vi "Lab Panel V2.5.vi"() -> ()   [LabVIEW 2013]
uses:
  <vilib>/Platform/TimedLoop/XDataNode/timing_clust.ctl
  <vilib>/Platform/TimedLoop/XDataNode/nitl_modes.ctl
  <vilib>/Platform/TimedLoop/XDataNode/wakeup.ctl
  <vilib>/platform/TimedLoop/XDataNode/XDataNode.xnode
  <vilib>/Platform/TimedLoop/XDataNode/XDNodeRunTimeDep.lvlib
panel:
  out "TEMP update":bool
  out "AI update":bool
  in  "stop":bool
  in  "Tab Control 2":T1(tab)
  out "LAB05-2 (SIG)":T2 {"PF" format="%.2f"; "AMPS" format="%.1f"}
  out "LAB05-1 (SIG)":T2 {"PF" format="%.2f"; "AMPS" format="%.1f"}
  out "LAB04-2 (SIG)":T2 {"PF" format="%.2f"; "AMPS" format="%.1f"}
  out "LAB04-1 (SIG)":T2 {"PF" format="%.2f"; "AMPS" format="%.1f"}
  out "LAB03-2 (SIG)":T2 {"PF" format="%.2f"; "AMPS" format="%.1f"}
  out "LAB03-1 (SIG)":T2 {"PF" format="%.2f"; "AMPS" format="%.1f"}
  out "LAB02-2 (SIG)":T2 {"PF" format="%.2f"; "AMPS" format="%.1f"}
  in  "LAB01-1RUN":bool
  in  "LAB05-1 (O/I)":bool
  in  "LAB05-2 (O/I)":bool
  in  "LAB04-1 (O/I)":bool
  in  "LAB04-2 (O/I)":bool
  in  "LAB02-1 (O/I)":bool
  in  "LAB02-2 (O/I)":bool
  in  "LAB01-2 (O/I)":bool
  in  "LAB01-1 (O/I)":bool
  in  "LAB03-1 (O/I)":bool
  in  "LAB05-2 RUN":bool
  in  "LAB05-1 RUN":bool
  in  "LAB04-2 RUN":bool
  in  "LAB04-1 RUN":bool
  in  "LAB03-2 RUN":bool
  in  "LAB03-1 RUN":bool
  in  "LAB02-2 RUN":bool
  in  "LAB02-1 RUN":bool
  in  "LAB01-2 RUN":bool
  in  "LAB05-2 SELECT":T3(radio)
  in  "LAB05-1 SELECT":T3(radio)
  in  "LAB04-2 SELECT":T3(radio)
  in  "LAB04-1 SELECT":T3(radio)
  in  "LAB03-2 SELECT":T3(radio)
  in  "LAB03-1 SELECT":T3(radio)
  in  "LAB02-2 SELECT":T3(radio)
  in  "LAB02-1 SELECT":T3(radio)
  in  "LAB01-2 SELECT":T3(radio)
  in  "LAB01-1 SELECT":T3(radio)
  in  "LAB03-2 (O/I)":bool
  out "LAB01-1 (SIG)":T2 {"PF" format="%.2f"; "AMPS" format="%.1f"}
  out "LAB01-2 (SIG)":T2 {"PF" format="%.2f"; "AMPS" format="%.1f"}
  out "LAB02-1 (SIG)":T2 {"PF" format="%.2f"; "AMPS" format="%.1f"}
  out "LAB05-2 (RESULT)":bool
  out "LAB05-1 (RESULT)":bool
  out "LAB04-2 (RESULT)":bool
  out "LAB04-1 (RESULT)":bool
  out "LAB03-2 (RESULT)":bool
  out "LAB03-1 (RESULT)":bool
  out "LAB02-2 (RESULT)":bool
  out "LAB02-1 (RESULT)":bool
  out "LAB01-2 (RESULT)":bool
  out "LAB01-1 (RESULT)":bool
  in  "LAB05 (SET)":T4={"1 Name"="", "1 Description"="", "1 (CYCLES)"=1.0, "1 (T-RISE mins)"=1.0, "1 (T-RISE deg C)"=1.0, "2 Name"="", "2 Description"="", "2 (CYCLES)"=1.0, "2 (T-RISE mins)"=1.0, "2 (T-RISE deg C)"=1.0} {"2 (T-RISE deg C)" min=1.0 max=100.0 step=1.0 format="%#.0f"; "2 (T-RISE mins)" min=0.0 max=1000.0 step=10.0 format="%#.0f"; "2 (CYCLES)" min=0.0 max=100000.0 step=10.0; "1 (T-RISE deg C)" min=1.0 max=100.0 step=1.0 format="%#.0f"; "1 (T-RISE mins)" min=0.0 max=1000.0 step=10.0 format="%#.0f"; "1 (CYCLES)" min=0.0 max=100000.0 step=10.0}
  in  "LAB04 (SET)":T4={"1 Name"="", "1 Description"="", "1 (CYCLES)"=1.0, "1 (T-RISE mins)"=1.0, "1 (T-RISE deg C)"=1.0, "2 Name"="", "2 Description"="", "2 (CYCLES)"=1.0, "2 (T-RISE mins)"=1.0, "2 (T-RISE deg C)"=1.0} {"2 (T-RISE deg C)" min=1.0 max=100.0 step=1.0 format="%#.0f"; "2 (T-RISE mins)" min=0.0 max=1000.0 step=10.0 format="%#.0f"; "2 (CYCLES)" min=0.0 max=100000.0 step=10.0; "1 (T-RISE deg C)" min=1.0 max=100.0 step=1.0 format="%#.0f"; "1 (T-RISE mins)" min=0.0 max=1000.0 step=10.0 format="%#.0f"; "1 (CYCLES)" min=0.0 max=100000.0 step=10.0}
  in  "LAB03 (SET)":T4={"1 Name"="", "1 Description"="", "1 (CYCLES)"=1.0, "1 (T-RISE mins)"=1.0, "1 (T-RISE deg C)"=1.0, "2 Name"="", "2 Description"="", "2 (CYCLES)"=1.0, "2 (T-RISE mins)"=1.0, "2 (T-RISE deg C)"=1.0} {"2 (T-RISE deg C)" min=1.0 max=100.0 step=1.0 format="%#.0f"; "2 (T-RISE mins)" min=0.0 max=1000.0 step=10.0 format="%#.0f"; "2 (CYCLES)" min=0.0 max=100000.0 step=10.0; "1 (T-RISE deg C)" min=1.0 max=100.0 step=1.0 format="%#.0f"; "1 (T-RISE mins)" min=0.0 max=1000.0 step=10.0 format="%#.0f"; "1 (CYCLES)" min=0.0 max=100000.0 step=10.0}
  out "LAB05 (DISP)":T5 {"2 (T-RISE min)" format="%#.0f"; "2 (CYCLE)" format="%#.0f"; "1 (T-RISE min)" format="%#.0f"; "1 (CYCLE)" format="%#.0f"}
  out "LAB04 (DISP)":T5 {"2 (T-RISE min)" format="%#.0f"; "2 (CYCLE)" format="%#.0f"; "1 (T-RISE min)" format="%#.0f"; "1 (CYCLE)" format="%#.0f"}
  out "LAB03 (DISP)":T5 {"2 (T-RISE min)" format="%#.0f"; "2 (CYCLE)" format="%#.0f"; "1 (T-RISE min)" format="%#.0f"; "1 (CYCLE)" format="%#.0f"}
  out "LAB02 (DISP)":T5 {"2 (T-RISE min)" format="%#.0f"; "2 (CYCLE)" format="%#.0f"; "1 (T-RISE min)" format="%#.0f"; "1 (CYCLE)" format="%#.0f"}
  in  "LAB02 (SET)":T4={"1 Name"="", "1 Description"="", "1 (CYCLES)"=1.0, "1 (T-RISE mins)"=1.0, "1 (T-RISE deg C)"=1.0, "2 Name"="", "2 Description"="", "2 (CYCLES)"=1.0, "2 (T-RISE mins)"=1.0, "2 (T-RISE deg C)"=1.0} {"2 (T-RISE deg C)" min=1.0 max=100.0 step=1.0 format="%#.0f"; "2 (T-RISE mins)" min=0.0 max=1000.0 step=10.0 format="%#.0f"; "2 (CYCLES)" min=0.0 max=100000.0 step=10.0; "1 (T-RISE deg C)" min=1.0 max=100.0 step=1.0 format="%#.0f"; "1 (T-RISE mins)" min=0.0 max=1000.0 step=10.0 format="%#.0f"; "1 (CYCLES)" min=0.0 max=100000.0 step=10.0}
  out "LAB01 (DISP)":T5 {"2 (T-RISE min)" format="%#.0f"; "2 (CYCLE)" format="%#.0f"; "1 (T-RISE min)" format="%.2f"; "1 (CYCLE)" format="%#.0f"}
  in  "LAB01 (SET)":T4={"1 Name"="", "1 Description"="", "1 (CYCLES)"=1.0, "1 (T-RISE mins)"=1.0, "1 (T-RISE deg C)"=1.0, "2 Name"="", "2 Description"="", "2 (CYCLES)"=1.0, "2 (T-RISE mins)"=1.0, "2 (T-RISE deg C)"=1.0} {"2 (T-RISE deg C)" min=1.0 max=100.0 step=1.0 format="%#.0f"; "2 (T-RISE mins)" min=1.0 max=1000.0 step=10.0 format="%#.0f"; "2 (CYCLES)" min=1.0 max=100000.0 step=10.0; "1 (T-RISE deg C)" min=1.0 max=100.0 step=1.0 format="%#.0f"; "1 (T-RISE mins)" min=1.0 max=1000.0 step=10.0 format="%#.0f"; "1 (CYCLES)" min=1.0 max=100000.0 step=10.0}
  out "LAB05 (TEMP START)":T6
  out "LAB04 (TEMP START)":T6
  out "LAB03 (TEMP START)":T6
  out "LAB02 (TEMP START)":T6
  out "LAB01 (TEMP START)":T6
  in  "JIG ON TIME (S)":dbl=1.0 min=1.0 max=10.0 step=0.5 format="%.1g"
  in  "JIG OFF TIME (S)":dbl=2.0 min=2.0 max=10.0 step=0.5 format="%.1g"
  out "LAB01-1 (JIG)":bool
  out "LAB01-2 (JIG)":bool
  out "LAB02-1 (JIG)":bool
  out "LAB02-2 (JIG)":bool
  out "LAB03-1 (JIG)":bool
  out "LAB03-2 (JIG)":bool
  out "LAB04-1 (JIG)":bool
  out "LAB04-2 (JIG)":bool
  out "LAB05-1 (JIG)":bool
  out "LAB05-2 (JIG)":bool
  out "LAB01 (CAL)":T7 {"2 (TN) cal" min=0.0 step=0.01 format="%.2f"; "2 (TL) cal" min=0.0 step=0.01 format="%.2f"; "2 (PF) cal" min=0.0 step=0.01 format="%.2f"; "2 (V) cal" min=0.0 step=0.01 format="%.2f"; "2 (A) cal" min=0.0 step=0.01 format="%.2f"; "1 (TN) cal" min=0.0 step=0.01 format="%.2f"; "1 (TL) cal" min=0.0 step=0.01 format="%.2f"; "1 (PF) cal" min=0.0 step=0.01 format="%.2f"; "1 (V) cal" min=0.0 step=0.01 format="%.2f"; "1  (A) cal" min=0.0 step=0.01 format="%.2f"}
  out "LAB03 (CAL)":T7 {"2 (TN) cal" min=0.0 step=0.01 format="%.2f"; "2 (TL) cal" min=0.0 step=0.01 format="%.2f"; "2 (PF) cal" min=0.0 step=0.01 format="%.2f"; "2 (V) cal" min=0.0 step=0.01 format="%.2f"; "2 (A) cal" min=0.0 step=0.01 format="%.2f"; "1 (TN) cal" min=0.0 step=0.01 format="%.2f"; "1 (TL) cal" min=0.0 step=0.01 format="%.2f"; "1 (PF) cal" min=0.0 step=0.01 format="%.2f"; "1 (V) cal" min=0.0 step=0.01 format="%.2f"; "1  (A) cal" min=0.0 step=0.01 format="%.2f"}
  out "LAB02 (CAL)":T8 {"2 (TN) cal" min=0.0 step=0.01 format="%.2f"; "2 (TL) cal" min=0.0 step=0.01 format="%.2f"; "2 (PF) cal" min=0.0 step=0.01 format="%.2f"; "2 (V) cal" min=0.0 step=0.01 format="%.2f"; "2 (A) cal" min=0.0 step=0.01 format="%.2f"; "1 (TN) cal" min=0.0 step=0.01 format="%.2f"; "1 (TL) cal" min=0.0 step=0.01 format="%.2f"; "1 (PF) cal" min=0.0 step=0.01 format="%.2f"; "1 (V) cal" min=0.0 step=0.01 format="%.2f"; "1 (A) cal" min=0.0 step=0.01 format="%.2f"}
  out "LAB05 (CAL)":T7 {"2 (TN) cal" min=0.0 step=0.01 format="%.2f"; "2 (TL) cal" min=0.0 step=0.01 format="%.2f"; "2 (PF) cal" min=0.0 step=0.01 format="%.2f"; "2 (V) cal" min=0.0 step=0.01 format="%.2f"; "2 (A) cal" min=0.0 step=0.01 format="%.2f"; "1 (TN) cal" min=0.0 step=0.01 format="%.2f"; "1 (TL) cal" min=0.0 step=0.01 format="%.2f"; "1 (PF) cal" min=0.0 step=0.01 format="%.2f"; "1 (V) cal" min=0.0 step=0.01 format="%.2f"; "1  (A) cal" min=0.0 step=0.01 format="%.2f"}
  out "LAB04 (CAL)":T7 {"2 (TN) cal" min=0.0 step=0.01 format="%.2f"; "2 (TL) cal" min=0.0 step=0.01 format="%.2f"; "2 (PF) cal" min=0.0 step=0.01 format="%.2f"; "2 (V) cal" min=0.0 step=0.01 format="%.2f"; "2 (A) cal" min=0.0 step=0.01 format="%.2f"; "1 (TN) cal" min=0.0 step=0.01 format="%.2f"; "1 (TL) cal" min=0.0 step=0.01 format="%.2f"; "1 (PF) cal" min=0.0 step=0.01 format="%.2f"; "1 (V) cal" min=0.0 step=0.01 format="%.2f"; "1  (A) cal" min=0.0 step=0.01 format="%.2f"}
  out "calibration file error out":errorcluster
  in  "CALIBRATE":bool
  in  "Tab Control":T9(tab)
  out "LAB01-2 (GRAPH)":dynamicdata(graph)
  out "LAB01-1 (GRAPH)":dynamicdata(graph)
  out "LAB02-2 (GRAPH)":dynamicdata(graph)
  out "LAB02-1 (GRAPH)":dynamicdata(graph)
  out "LAB03-2 (GRAPH)":dynamicdata(graph)
  out "LAB03-1 (GRAPH)":dynamicdata(graph)
  out "LAB04-2 (GRAPH)":dynamicdata(graph)
  out "LAB04-1 (GRAPH)":dynamicdata(graph)
  out "LAB05-2 (GRAPH)":dynamicdata(graph)
  out "LAB05-1 (GRAPH)":dynamicdata(graph)
  out "LAB05 TEMP":T10
  out "LAB04 TEMP":T10
  out "LAB02 TEMP":T10
  out "LAB01 TEMP":T10
  out "LAB03 TEMP":T10
  out "Analog Error Array":errorcluster[](array[cluster])
  out "AI loop time":dbl format="%.6g"
  out "loops":dbl
  in  "loop  delay(mS)":dbl
  out "on loops":dbl
  out "off loops":dbl
  out "jig cycle":dbl
  out "LAB01-1 (TDMS)":refnum<k34>
  out "data file error":errorcluster
  out "LAB01-2 (TDMS)":refnum<k34>
  out "LAB02-1 (TDMS)":refnum<k34>
  out "LAB02-2 (TDMS)":refnum<k34>
  out "LAB03-1 (TDMS)":refnum<k34>
  out "LAB03-2 (TDMS)":refnum<k34>
  out "LAB04-1 (TDMS)":refnum<k34>
  out "LAB04-2 (TDMS)":refnum<k34>
  out "LAB05-1 (TDMS)":refnum<k34>
  out "LAB05-2 (TDMS)":refnum<k34>
  # "LAB01"
  # "LAB02"
  # "LAB05"
  # "LAB03"
  # "LAB04"
  # "LAB01"
  # "LAB02"
  # "LAB03"
  # "LAB04"
  # "LAB05"
  # "JIG SET"
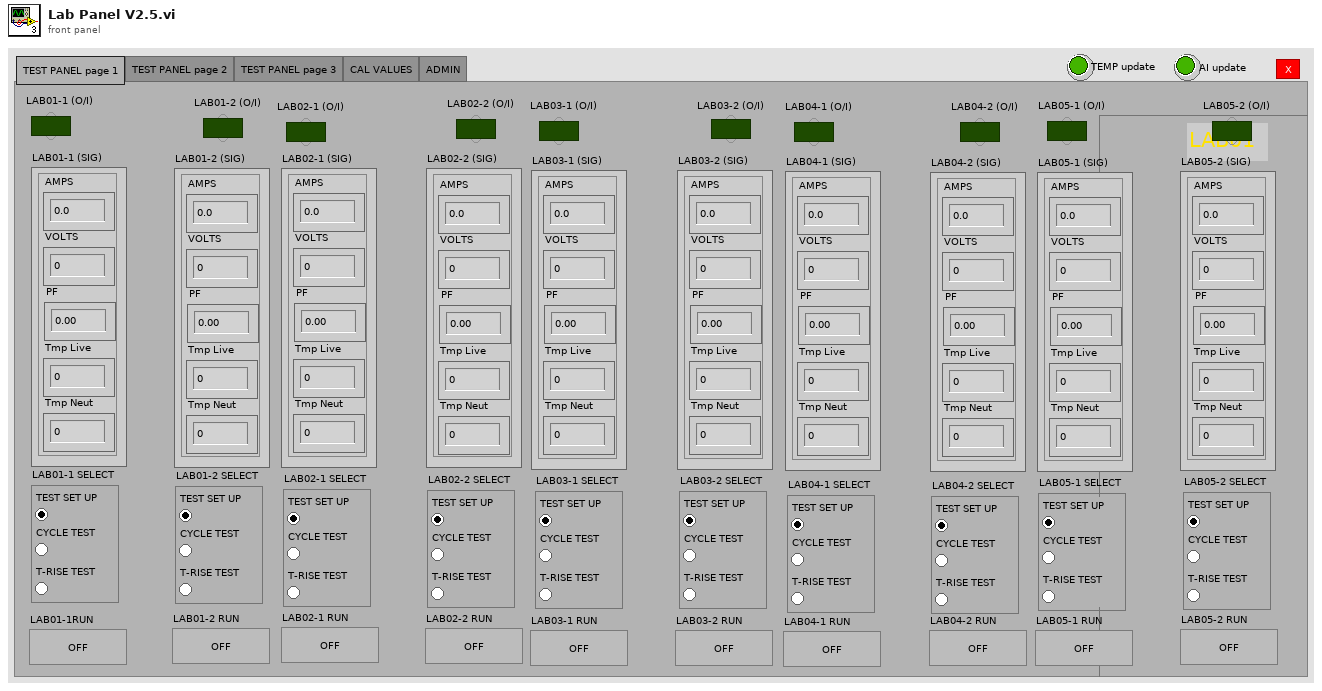
[diagram p1: front panel]
types:
  T1 = enum32{"TEST PANEL page 1", "TEST PANEL page 2", "TEST PANEL page 3", "CAL VALUES", "ADMIN"}
  T2 = cluster{"AMPS":dbl, "VOLTS":dbl, "PF":dbl, "Tmp Live":dbl, "Tmp Neut":dbl}
  T3 = enum32{"TEST SET UP", "CYCLE TEST", "T-RISE TEST"}
  T4 = cluster{"1 Name":string, "1 Description":string, "1 (CYCLES)":dbl, "1 (T-RISE mins)":dbl, "1 (T-RISE deg C)":dbl, "2 Name":string, "2 Description":string, "2 (CYCLES)":dbl, "2 (T-RISE mins)":dbl, "2 (T-RISE deg C)":dbl}
  T5 = cluster{"1 (CYCLE)":dbl, "1 (T-RISE min)":dbl, "1 (STATUS)":string, "2 (CYCLE)":dbl, "2 (T-RISE min)":dbl, "2 (STATUS)":string}
  T6 = cluster{"1 (TL)":dbl, "1 (TN)":dbl, "2 (TL)":dbl, "2 (TN)":dbl}
  T7 = cluster{"1  (A) cal":dbl, "1 (V) cal":dbl, "1 (PF) cal":dbl, "1 (TL) cal":dbl, "1 (TN) cal":dbl, "2 (A) cal":dbl, "2 (V) cal":dbl, "2 (PF) cal":dbl, "2 (TL) cal":dbl, "2 (TN) cal":dbl}
  T8 = cluster{"1 (A) cal":dbl, "1 (V) cal":dbl, "1 (PF) cal":dbl, "1 (TL) cal":dbl, "1 (TN) cal":dbl, "2 (A) cal":dbl, "2 (V) cal":dbl, "2 (PF) cal":dbl, "2 (TL) cal":dbl, "2 (TN) cal":dbl}
  T9 = enum32{"LAB01", "LAB02", "LAB03", "LAB04", "LAB05", "TEMPERATURE", "ERROR"}
  T10 = cluster{"T1 Live":dbl, "T1 Neut":dbl, "T2 Live":dbl, "T2 Neut":dbl, "ID":dbl, "ER":dbl}
  T11 = typedef "XDNodeRunTimeDep.lvlib/timing_clust.ctl" = cluster{"Expected End [f-1]":u64, "Actual End [f-1]":u64, "Finished Late? [f-1]":bool, "Expected End [i-1]":u64, "Actual End [i-1]":u64, "Finished Late? [i-1]":bool, "Expected Start [i]":u64, "Actual Start [i]":u64, "Expected Start [f]":u64, "Actual Start [f]":u64, "Source Name":string, "Structure Name":string, "Period":i64, "Deadline":i64, "Offset":i64, "Start":i64, "Priority":i32, "Timeout":i32, "Mode":T12, "Wakeup Reason":T13, "Error":errorcluster, "Source Type":string, "Secondary Source Type":string, "Global End Time":u64, "Global Start Time":u64, "Frame Duration":u64, "Iteration Duration":u64, "Assigned CPU":i32, "I/O Scan Engine Mode":u32}
  T12 = typedef "XDNodeRunTimeDep.lvlib/nitl_modes.ctl" = enum32{"No Change", "Process missed periods, maintain original phase", "Discard missed periods, maintain original phase", "Process missed periods, ignore original phase", "Discard missed periods, ignore original phase"}
  T13 = typedef "XDNodeRunTimeDep.lvlib/wakeup.ctl" = enum32{"Normal", "Aborted", "Asynchronous wakeup", "Timing source error", "Timed loop error", "Timeout"}
  T14 = enum16{"open", "open or create", "create or replace", "create", "open (read-only)"}
  T15 = cluster{"T1":dbl, "T2":dbl, "T3":dbl, "T4":dbl, "ID":dbl, "ER":dbl}
  T16 = cluster{"LAB01-1 (A)":dbl, "LAB01-1 (V)":dbl, "LAB01-1 (PF)":dbl, "LAB01-2 (A)":dbl, "LAB01-2 (V)":dbl, "LAB01-2 (PF)":dbl}
  T17 = cluster{"LAB02-1 (A)":dbl, "LAB02-1 (V)":dbl, "LAB02-1 (PF)":dbl, "LAB02-2 (A)":dbl, "LAB02-2 (V)":dbl, "LAB02-2 (PF)":dbl}
  T18 = cluster{"LAB03-1 (A)":dbl, "LAB03-1 (V)":dbl, "LAB03-1 (PF)":dbl, "LAB03-2 (A)":dbl, "LAB03-2 (V)":dbl, "LAB03-2 (PF)":dbl}
  T19 = cluster{"LAB04-1 (A)":dbl, "LAB04-1 (V)":dbl, "LAB04-1 (PF)":dbl, "LAB04-2 (A)":dbl, "LAB04-2 (V)":dbl, "LAB04-2 (PF)":dbl}
  T20 = cluster{"LAB05-1 (A)":dbl, "LAB05-1 (V)":dbl, "LAB05-1 (PF)":dbl, "LAB05-2 (A)":dbl, "LAB05-2 (V)":dbl, "LAB05-2 (PF)":dbl}
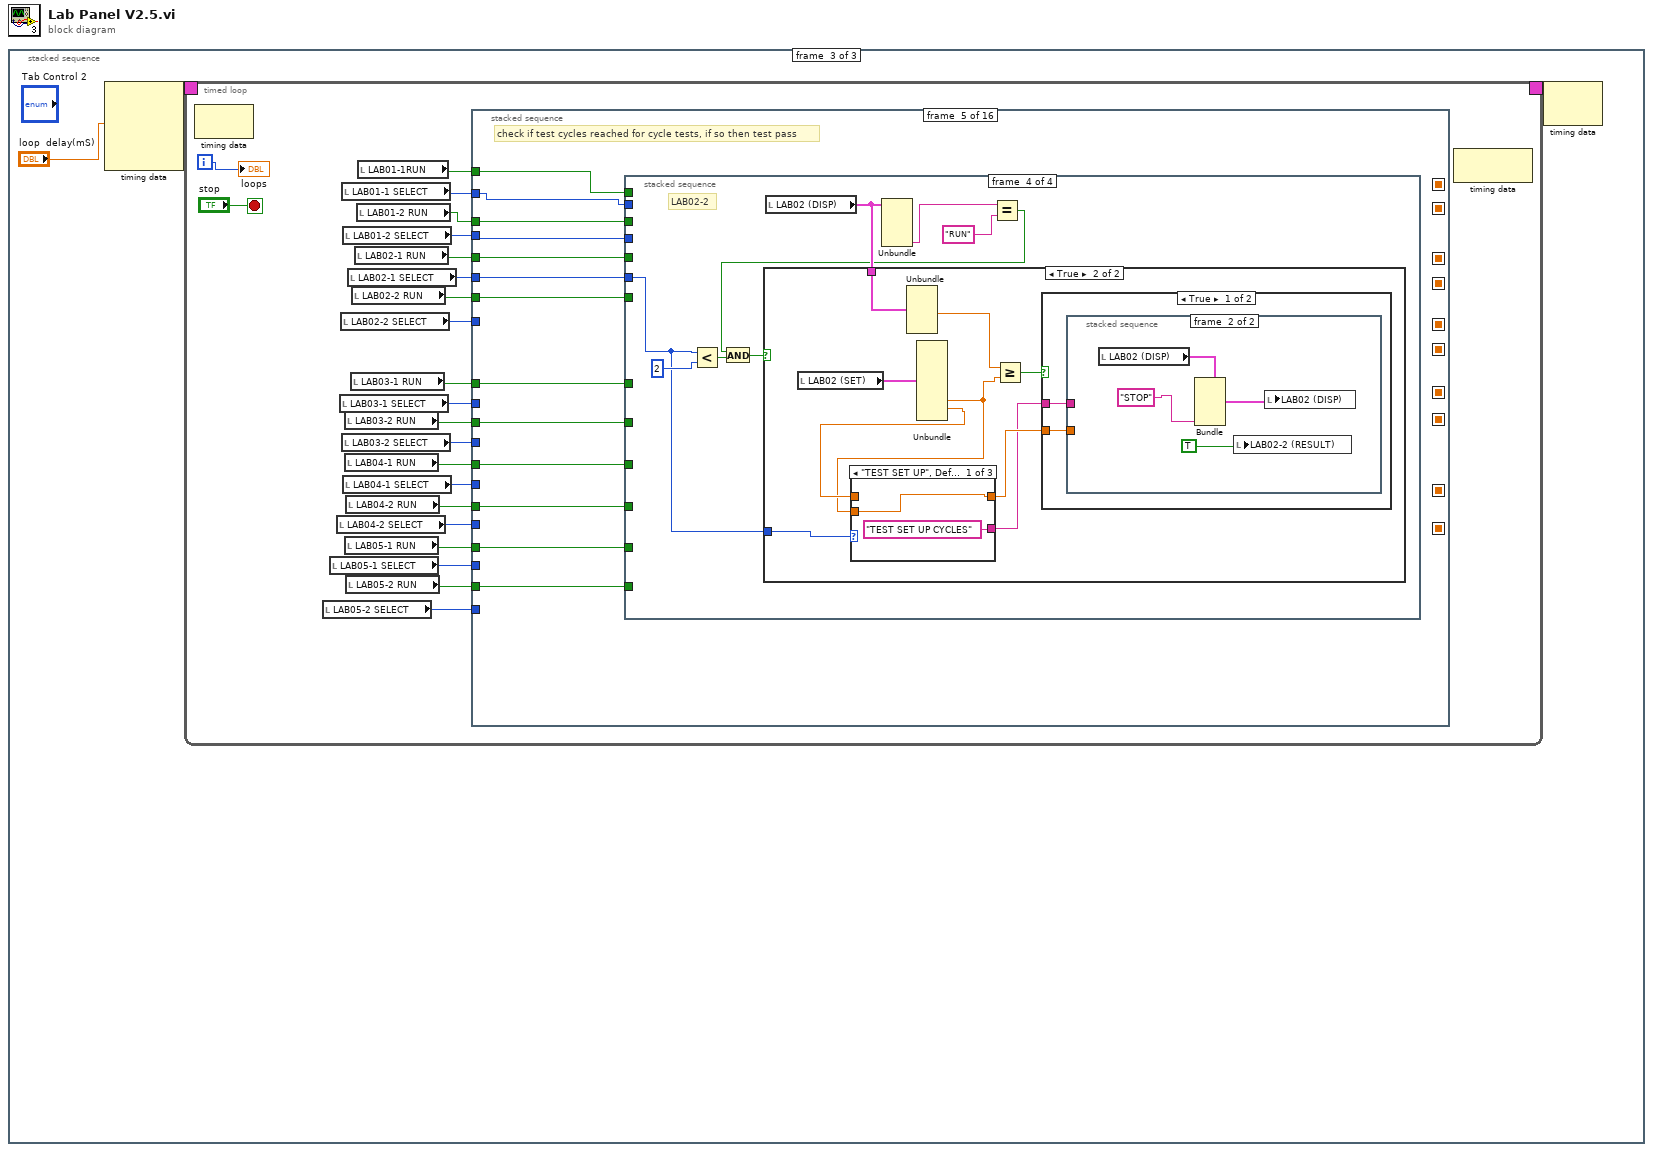
[diagram p0: block diagram]
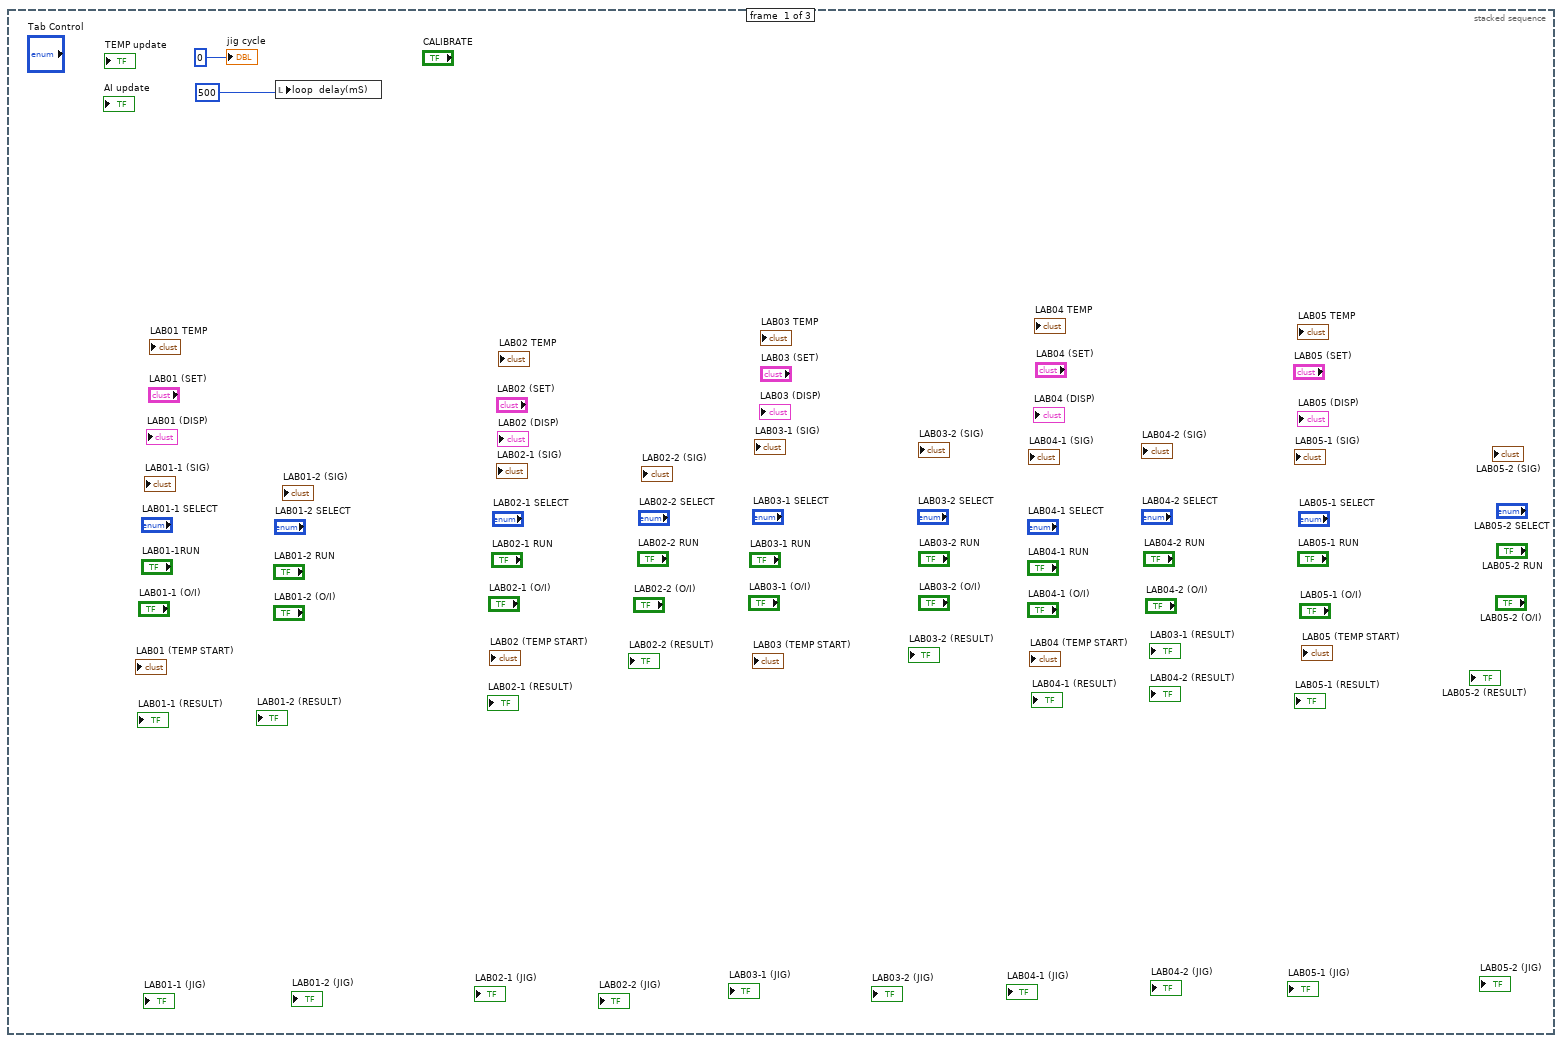
[diagram p2: hidden frame]
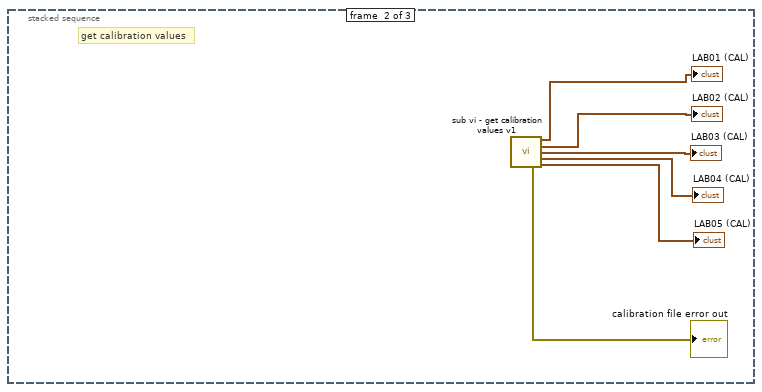
[diagram p3: hidden frame]
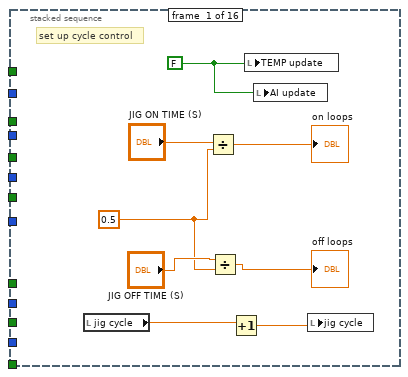
[diagram p4: hidden frame]
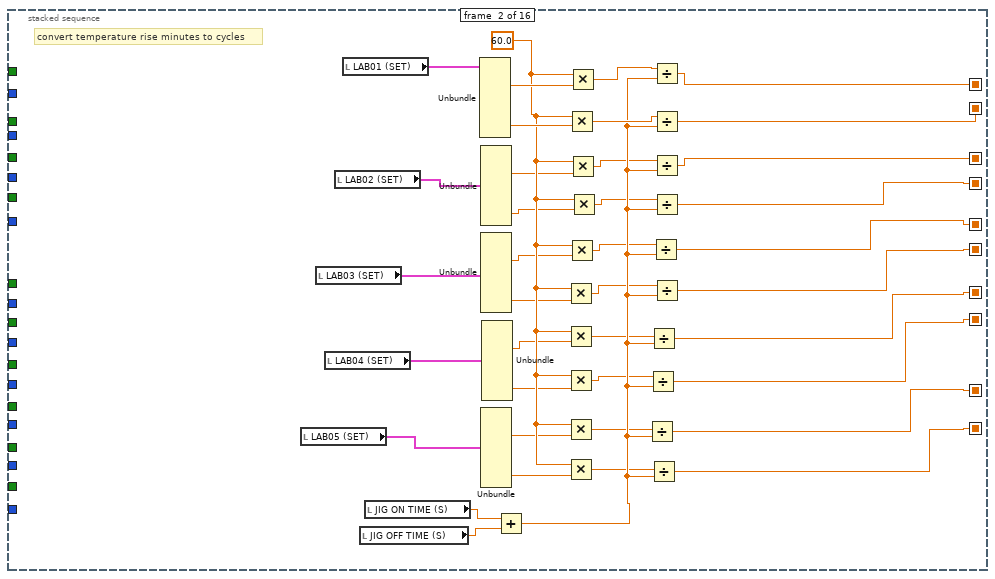
[diagram p5: hidden frame]
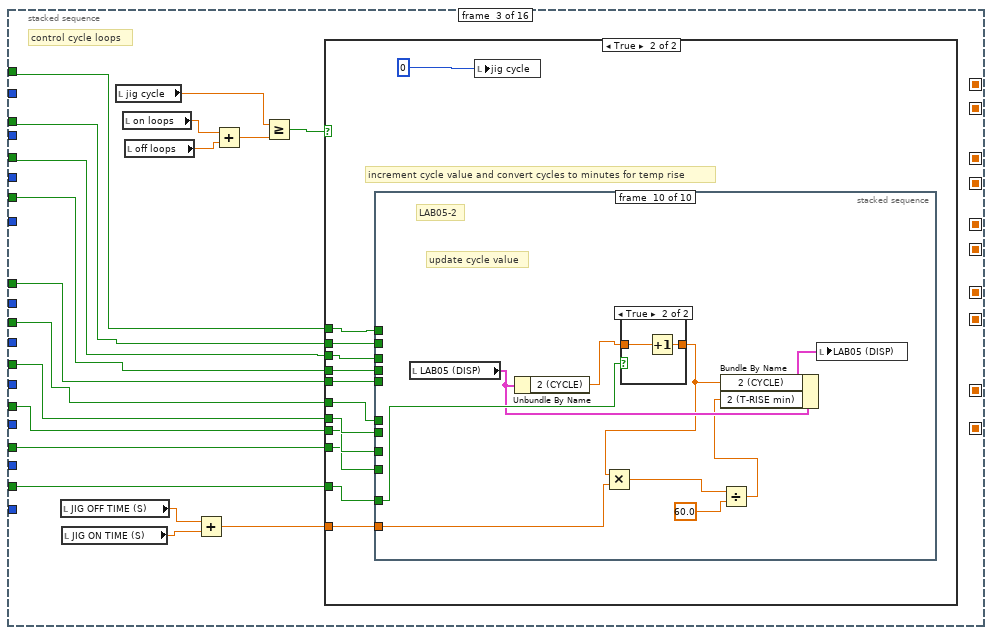
[diagram p6: hidden frame]
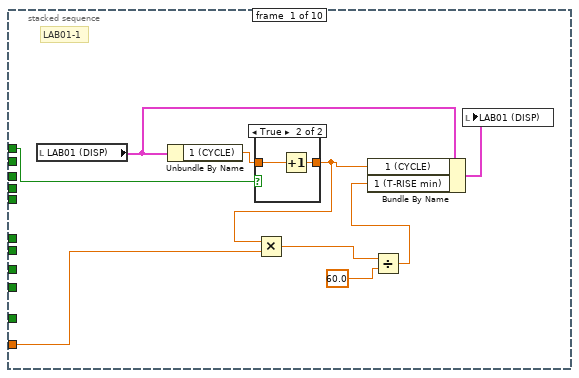
[diagram p8: hidden frame]
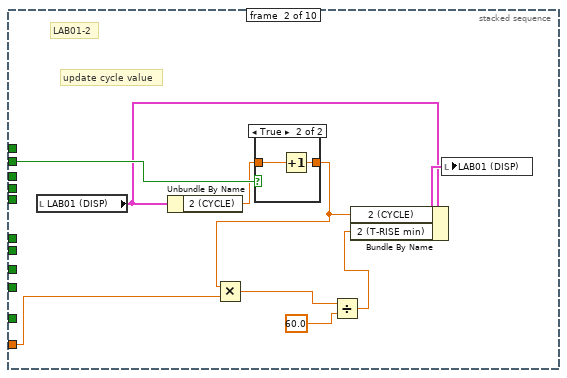
[diagram p10: hidden frame]
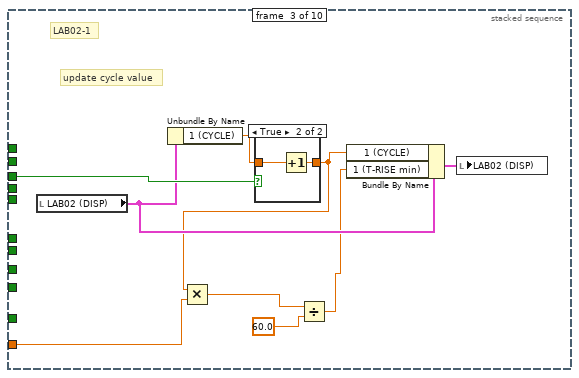
[diagram p12: hidden frame]
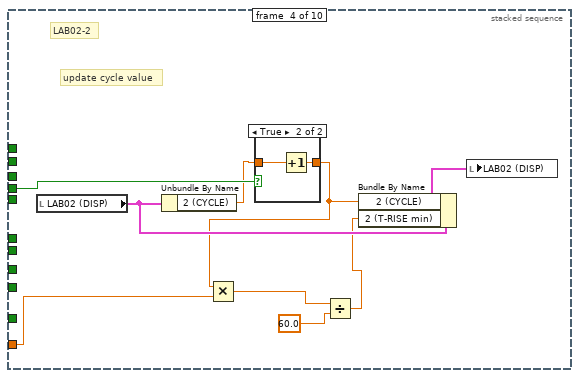
[diagram p14: hidden frame]
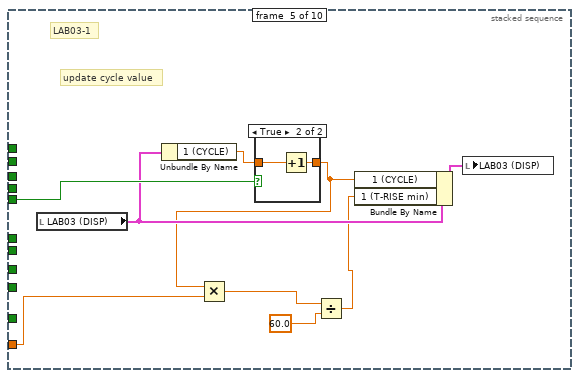
[diagram p16: hidden frame]
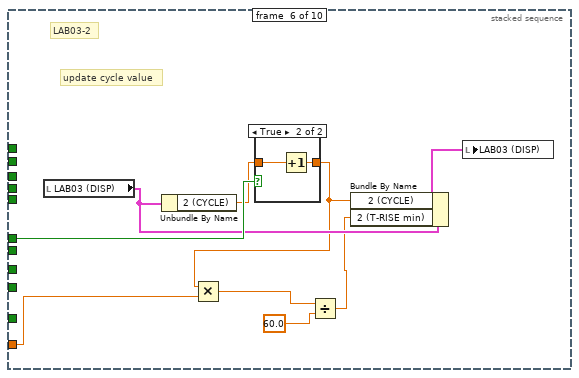
[diagram p18: hidden frame]
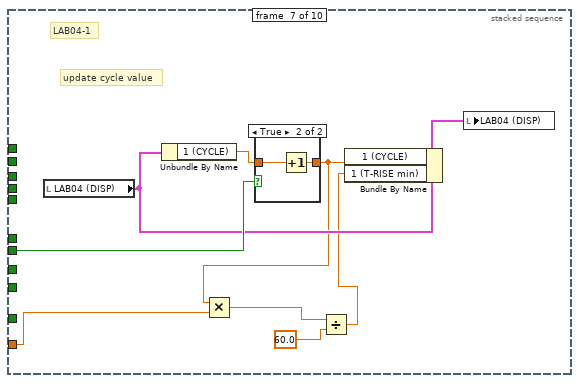
[diagram p20: hidden frame]
diagram:
  n1 = stacked-sequence {
    frame #0 {
      n2 = local write "loop  delay(mS)"(500) -> ()
      "jig cycle" <- 0
    }
    frame #1 {
      # "get calibration values"
      n3 = call "sub vi - get calibration values v1.vi"() -> ("LAB01 (CAL)"=→"LAB01 (CAL)":T7, "LAB02 (CAL)"=→"LAB02 (CAL)":T8, "LAB03 (CAL)"=→"LAB03 (CAL)":T7, "LAB04 (CAL)"=→"LAB04 (CAL)":T7, "calibration file error out"=→"calibration file error out":errorcluster, "LAB05 (CAL)"=→"LAB05 (CAL)":T7)  [unwired: 10 in]
    }
    frame #2 {
      n4 = node-c288("loop  delay(mS)") -> (w11:T11)  [unwired: 3 in]
      n5 = timed-loop {
        timing: w11 -> [_]
        timing-out: [_] -> w10
        i -> [w33]
        stop <- "stop" stop-if-true
        n6 = node-c288() -> ()  [unwired: 1 in, 1 out]
        n7 = local read "LAB05-2 SELECT"() -> (w12:T3)
        n8 = local read "LAB05-1 SELECT"() -> (w13:T3)
        n9 = local read "LAB04-2 SELECT"() -> (w14:T3)
        n10 = local read "LAB03-1 SELECT"() -> (w17:T3)
        n11 = local read "LAB02-2 SELECT"() -> (w18:T3)
        n12 = local read "LAB01-1 SELECT"() -> (w21:T3)
        n13 = local read "LAB03-2 SELECT"() -> (w16:T3)
        n14 = local read "LAB01-2 SELECT"() -> (w20:T3)
        n15 = local read "LAB04-1 SELECT"() -> (w15:T3)
        n16 = local read "LAB03-2 RUN"() -> (w26:bool)
        n17 = local read "LAB04-1 RUN"() -> (w25:bool)
        n18 = local read "LAB05-1 RUN"() -> (w23:bool)
        n19 = local read "LAB04-2 RUN"() -> (w24:bool)
        n20 = local read "LAB05-2 RUN"() -> (w22:bool)
        n21 = local read "LAB02-1 SELECT"() -> (w19:T3)
        n22 = local read "LAB03-1 RUN"() -> (w27:bool)
        n23 = local read "LAB02-2 RUN"() -> (w28:bool)
        n24 = local read "LAB02-1 RUN"() -> (w29:bool)
        n25 = local read "LAB01-2 RUN"() -> (w30:bool)
        n26 = local read "LAB01-1RUN"() -> (w31:bool)
        n27 = stacked-sequence {
          seq-local: [_ w79 _ _ _ _ _ _ _ _ _ _ _ _ _ _] -> [_ _ _ _ _ w1197 _ _ _ _ _ _ _ _ _ _]
          seq-local: [_ w78 _ _ _ _ _ _ _ _ _ _ _ _ _ _] -> [_ _ _ _ _ _ _ _ _ _ _ _ _ _ _ _]
          seq-local: [_ w51 _ _ _ _ _ _ _ _ _ _ _ _ _ _] -> [_ _ _ _ _ _ _ _ _ _ _ _ _ _ _ _]
          seq-local: [_ w50 _ _ _ _ _ _ _ _ _ _ _ _ _ _] -> [_ _ _ _ _ _ _ _ _ _ _ _ _ _ _ _]
          seq-local: [_ w49 _ _ _ _ _ _ _ _ _ _ _ _ _ _] -> [_ _ _ _ _ _ _ _ _ _ _ _ _ _ _ _]
          seq-local: [_ w48 _ _ _ _ _ _ _ _ _ _ _ _ _ _] -> [_ _ _ _ _ _ _ _ _ _ _ _ _ _ _ _]
          seq-local: [_ w47 _ _ _ _ _ _ _ _ _ _ _ _ _ _] -> [_ _ _ _ _ _ _ _ _ _ _ _ _ _ _ _]
          seq-local: [_ w46 _ _ _ _ _ _ _ _ _ _ _ _ _ _] -> [_ _ _ _ _ _ _ _ _ _ _ _ _ _ _ _]
          seq-local: [_ w45 _ _ _ _ _ _ _ _ _ _ _ _ _ _] -> [_ _ _ _ _ _ _ _ _ _ _ _ _ _ _ _]
          seq-local: [_ w44 _ _ _ _ _ _ _ _ _ _ _ _ _ _] -> [_ _ _ _ _ _ _ _ _ _ _ _ _ _ _ _]
          tunnel: w31 -> [_ _ w96 w252 w1052 w1208 w1245 _ _ _ _ _ w1681 w1737 w1796 _]
          tunnel: w30 -> [_ _ w95 w250 w1051 w1207 w1244 _ _ _ _ _ _ _ _ _]
          tunnel: w29 -> [_ _ w94 w248 w1050 w1206 w1243 _ _ _ _ _ _ _ _ _]
          tunnel: w28 -> [_ _ w93 w246 w1049 w1205 w1242 _ _ _ _ _ _ _ _ _]
          tunnel: w27 -> [_ _ w92 w244 w1048 w1204 w1241 _ _ _ _ _ _ _ _ _]
          tunnel: w26 -> [_ _ w91 w242 w1047 w1203 w1240 _ _ _ _ _ _ _ _ _]
          tunnel: w25 -> [_ _ w90 w240 w1046 w1202 w1239 _ _ _ _ _ _ _ _ _]
          tunnel: w24 -> [_ _ w89 w238 w1045 w1201 w1238 _ _ _ _ _ _ _ _ _]
          tunnel: w23 -> [_ _ w88 w236 w1044 w1200 w1237 _ _ _ _ _ _ _ _ _]
          tunnel: w22 -> [_ _ w87 w234 w1043 w1199 w1236 _ _ _ _ _ _ _ _ _]
          tunnel: w21 -> [_ _ _ w251 w1042 w1198 _ _ _ _ _ _ _ w1739 w1797 _]
          tunnel: w20 -> [_ _ _ w249 w1041 _ _ _ _ _ _ _ _ _ _ _]
          tunnel: w19 -> [_ _ _ w247 w1040 _ _ _ _ _ _ _ _ _ _ _]
          tunnel: w18 -> [_ _ _ w245 _ _ _ _ _ _ _ _ _ _ _ _]
          tunnel: w17 -> [_ _ _ w243 _ _ _ _ _ _ _ _ _ _ _ _]
          tunnel: w16 -> [_ _ _ w241 _ _ _ _ _ _ _ _ _ _ _ _]
          tunnel: w15 -> [_ _ _ w239 _ _ _ _ _ _ _ _ _ _ _ _]
          tunnel: w14 -> [_ _ _ w237 _ _ _ _ _ _ _ _ _ _ _ _]
          tunnel: w13 -> [_ _ _ w235 _ _ _ _ _ _ _ _ _ _ _ _]
          tunnel: w12 -> [_ _ _ w233 _ _ _ _ _ _ _ _ _ _ _ _]
          frame #0 {
            w36 = FALSE
            w41 = 0.5
            # "set up cycle control"
            n28 = local read "jig cycle"() -> (w40:dbl)
            n29 = Divide(x="JIG ON TIME (S)", y=w41) -> (x/y=→"on loops":dbl)
            n30 = Divide(x="JIG OFF TIME (S)", y=w41) -> (x/y=→"off loops":dbl)
            n31 = Increment(x=w40) -> (x+1=w39:dbl)
            n32 = local write "TEMP update"(w36) -> ()
            n33 = local write "AI update"(w36) -> ()
            n34 = local write "jig cycle"(w39) -> ()
          }
          frame #1 {
            w69 = 60.0
            # "convert temperature rise minutes to cycles"
            n35 = local read "LAB05 (SET)"() -> (w70:T4)
            n36 = local read "LAB03 (SET)"() -> (w72:T4)
            n37 = local read "LAB04 (SET)"() -> (w71:T4)
            n38 = local read "LAB02 (SET)"() -> (w73:T4)
            n39 = local read "LAB01 (SET)"() -> (w82:T4)
            n40 = local read "JIG OFF TIME (S)"() -> (w80:dbl)
            n41 = local read "JIG ON TIME (S)"() -> (w81:dbl)
            n42 = Unbundle(w82) -> ("1 (T-RISE mins)"=w77:dbl, "2 (T-RISE mins)"=w76:dbl)  [unwired: 8 out]
            n43 = Unbundle(w73) -> ("1 (T-RISE mins)"=w68:dbl, "2 (T-RISE mins)"=w67:dbl)  [unwired: 8 out]
            n44 = Unbundle(w72) -> ("1 (T-RISE mins)"=w66:dbl, "2 (T-RISE mins)"=w65:dbl)  [unwired: 8 out]
            n45 = Unbundle(w70) -> ("1 (T-RISE mins)"=w62:dbl, "2 (T-RISE mins)"=w61:dbl)  [unwired: 8 out]
            n46 = Unbundle(w71) -> ("1 (T-RISE mins)"=w64:dbl, "2 (T-RISE mins)"=w63:dbl)  [unwired: 8 out]
            n47 = Add(x=w81, y=w80) -> (x+y=w60:dbl)
            n48 = Multiply(x=w69, y=w65) -> (x*y=w56:dbl)
            n49 = Multiply(x=w69, y=w64) -> (x*y=w55:dbl)
            n50 = Multiply(x=w69, y=w63) -> (x*y=w54:dbl)
            n51 = Multiply(x=w69, y=w62) -> (x*y=w53:dbl)
            n52 = Multiply(x=w69, y=w61) -> (x*y=w52:dbl)
            n53 = Multiply(x=w69, y=w76) -> (x*y=w74:dbl)
            n54 = Multiply(x=w69, y=w66) -> (x*y=w57:dbl)
            n55 = Multiply(x=w69, y=w77) -> (x*y=w75:dbl)
            n56 = Multiply(x=w69, y=w68) -> (x*y=w59:dbl)
            n57 = Multiply(x=w69, y=w67) -> (x*y=w58:dbl)
            n58 = Divide(x=w53, y=w60) -> (x/y=w45:dbl)
            n59 = Divide(x=w54, y=w60) -> (x/y=w46:dbl)
            n60 = Divide(x=w55, y=w60) -> (x/y=w47:dbl)
            n61 = Divide(x=w52, y=w60) -> (x/y=w44:dbl)
            n62 = Divide(x=w57, y=w60) -> (x/y=w49:dbl)
            n63 = Divide(x=w75, y=w60) -> (x/y=w79:dbl)
            n64 = Divide(x=w74, y=w60) -> (x/y=w78:dbl)
            n65 = Divide(x=w59, y=w60) -> (x/y=w51:dbl)
            n66 = Divide(x=w58, y=w60) -> (x/y=w50:dbl)
            n67 = Divide(x=w56, y=w60) -> (x/y=w48:dbl)
          }
          frame #2 {
            # "control cycle loops"
            n68 = local read "JIG OFF TIME (S)"() -> (w85:dbl)
            n69 = local read "JIG ON TIME (S)"() -> (w84:dbl)
            n70 = local read "jig cycle"() -> (w98:dbl)
            n71 = local read "on loops"() -> (w100:dbl)
            n72 = local read "off loops"() -> (w99:dbl)
            n73 = Add(x=w85, y=w84) -> (x+y=w83:dbl)
            n74 = Add(x=w100, y=w99) -> (x+y=w86:dbl)
            n75 = Greater Or Equal?(x=w98, y=w86) -> (x >= y?=w97:bool)
            n76 = case shown="True" w97 {
              tunnel: w96 -> [_ w111]
              tunnel: w95 -> [_ w110]
              tunnel: w94 -> [_ w109]
              tunnel: w93 -> [_ w108]
              tunnel: w92 -> [_ w107]
              tunnel: w91 -> [_ w106]
              tunnel: w90 -> [_ w105]
              tunnel: w89 -> [_ w104]
              tunnel: w88 -> [_ w103]
              tunnel: w87 -> [_ w102]
              tunnel: w83 -> [_ w101]
              frame False {
              }
              frame True {
                # "increment cycle value and convert cycles to minutes for temp rise"
                n77 = stacked-sequence {
                  tunnel: w111 -> [w121 _ _ _ _ _ _ _ _ _]
                  tunnel: w110 -> [_ w133 _ _ _ _ _ _ _ _]
                  tunnel: w109 -> [_ _ w145 _ _ _ _ _ _ _]
                  tunnel: w108 -> [_ _ _ w157 _ _ _ _ _ _]
                  tunnel: w107 -> [_ _ _ _ w169 _ _ _ _ _]
                  tunnel: w106 -> [_ _ _ _ _ w181 _ _ _ _]
                  tunnel: w105 -> [_ _ _ _ _ _ w193 _ _ _]
                  tunnel: w104 -> [_ _ _ _ _ _ _ w205 _ _]
                  tunnel: w103 -> [_ _ _ _ _ _ _ _ w217 _]
                  tunnel: w102 -> [_ _ _ _ _ _ _ _ _ w229]
                  tunnel: w101 -> [w113 w127 w139 w151 w163 w175 w187 w199 w211 w223]
                  frame #0 {
                    # "LAB01-1"
                    n78 = local read "LAB01 (DISP)"() -> (w118:T5)
                    n79 = Unbundle By Name(w118) -> ("1 (CYCLE)"=w119:dbl)
                    n80 = case shown="True" w121 {
                      tunnel: w119 -> [w122 w124]
                      tunnel: [w122 w123] -> w115
                      frame False {
                      }
                      frame True {
                        n81 = Increment(x=w124) -> (x+1=w123:dbl)
                      }
                    }
                    n82 = Multiply(x=w115, y=w113) -> (x*y=w114:dbl)
                    n83 = Divide(x=w114, y=60.0) -> (x/y=w116:dbl)
                    n84 = Bundle By Name(cluster=w118, "1 (CYCLE)"=w115, "1 (T-RISE min)"=w116) -> (w120:T5)
                    n85 = local write "LAB01 (DISP)"(w120) -> ()
                  }
                  frame #1 {
                    # "update cycle value"
                    # "LAB01-2"
                    n86 = local read "LAB01 (DISP)"() -> (w131:T5)
                    n87 = Unbundle By Name(w131) -> ("2 (CYCLE)"=w130:dbl)
                    n88 = case shown="True" w133 {
                      tunnel: w130 -> [w134 w136]
                      tunnel: [w134 w135] -> w126
                      frame False {
                      }
                      frame True {
                        n89 = Increment(x=w136) -> (x+1=w135:dbl)
                      }
                    }
                    n90 = Multiply(x=w126, y=w127) -> (x*y=w128:dbl)
                    n91 = Divide(x=w128, y=60.0) -> (x/y=w125:dbl)
                    n92 = Bundle By Name(cluster=w131, "2 (CYCLE)"=w126, "2 (T-RISE min)"=w125) -> (w132:T5)
                    n93 = local write "LAB01 (DISP)"(w132) -> ()
                  }
                  frame #2 {
                    # "update cycle value"
                    # "LAB02-1"
                    n94 = local read "LAB02 (DISP)"() -> (w143:T5)
                    n95 = Unbundle By Name(w143) -> ("1 (CYCLE)"=w142:dbl)
                    n96 = case shown="True" w145 {
                      tunnel: [w146 w148] -> w138
                      tunnel: w142 -> [w146 w147]
                      frame False {
                      }
                      frame True {
                        n97 = Increment(x=w147) -> (x+1=w148:dbl)
                      }
                    }
                    n98 = Multiply(x=w138, y=w139) -> (x*y=w140:dbl)
                    n99 = Divide(x=w140, y=60.0) -> (x/y=w137:dbl)
                    n100 = Bundle By Name(cluster=w143, "1 (CYCLE)"=w138, "1 (T-RISE min)"=w137) -> (w144:T5)
                    n101 = local write "LAB02 (DISP)"(w144) -> ()
                  }
                  frame #3 {
                    # "update cycle value"
                    # "LAB02-2"
                    n102 = local read "LAB02 (DISP)"() -> (w155:T5)
                    n103 = Unbundle By Name(w155) -> ("2 (CYCLE)"=w154:dbl)
                    n104 = case shown="True" w157 {
                      tunnel: [w158 w160] -> w150
                      tunnel: w154 -> [w158 w159]
                      frame False {
                      }
                      frame True {
                        n105 = Increment(x=w159) -> (x+1=w160:dbl)
                      }
                    }
                    n106 = Multiply(x=w150, y=w151) -> (x*y=w152:dbl)
                    n107 = Divide(x=w152, y=60.0) -> (x/y=w149:dbl)
                    n108 = Bundle By Name(cluster=w155, "2 (CYCLE)"=w150, "2 (T-RISE min)"=w149) -> (w156:T5)
                    n109 = local write "LAB02 (DISP)"(w156) -> ()
                  }
                  frame #4 {
                    # "update cycle value"
                    # "LAB03-1"
                    n110 = local read "LAB03 (DISP)"() -> (w167:T5)
                    n111 = Unbundle By Name(w167) -> ("1 (CYCLE)"=w166:dbl)
                    n112 = case shown="True" w169 {
                      tunnel: [w170 w172] -> w162
                      tunnel: w166 -> [w170 w171]
                      frame False {
                      }
                      frame True {
                        n113 = Increment(x=w171) -> (x+1=w172:dbl)
                      }
                    }
                    n114 = Multiply(x=w162, y=w163) -> (x*y=w164:dbl)
                    n115 = Divide(x=w164, y=60.0) -> (x/y=w161:dbl)
                    n116 = Bundle By Name(cluster=w167, "1 (CYCLE)"=w162, "1 (T-RISE min)"=w161) -> (w168:T5)
                    n117 = local write "LAB03 (DISP)"(w168) -> ()
                  }
                  frame #5 {
                    # "update cycle value"
                    # "LAB03-2"
                    n118 = local read "LAB03 (DISP)"() -> (w179:T5)
                    n119 = Unbundle By Name(w179) -> ("2 (CYCLE)"=w178:dbl)
                    n120 = case shown="True" w181 {
                      tunnel: [w182 w184] -> w174
                      tunnel: w178 -> [w182 w183]
                      frame False {
                      }
                      frame True {
                        n121 = Increment(x=w183) -> (x+1=w184:dbl)
                      }
                    }
                    n122 = Multiply(x=w174, y=w175) -> (x*y=w176:dbl)
                    n123 = Divide(x=w176, y=60.0) -> (x/y=w173:dbl)
                    n124 = Bundle By Name(cluster=w179, "2 (CYCLE)"=w174, "2 (T-RISE min)"=w173) -> (w180:T5)
                    n125 = local write "LAB03 (DISP)"(w180) -> ()
                  }
                  frame #6 {
                    # "update cycle value"
                    # "LAB04-1"
                    n126 = local read "LAB04 (DISP)"() -> (w191:T5)
                    n127 = Unbundle By Name(w191) -> ("1 (CYCLE)"=w190:dbl)
                    n128 = case shown="True" w193 {
                      tunnel: [w194 w196] -> w186
                      tunnel: w190 -> [w194 w195]
                      frame False {
                      }
                      frame True {
                        n129 = Increment(x=w195) -> (x+1=w196:dbl)
                      }
                    }
                    n130 = Multiply(x=w186, y=w187) -> (x*y=w188:dbl)
                    n131 = Divide(x=w188, y=60.0) -> (x/y=w185:dbl)
                    n132 = Bundle By Name(cluster=w191, "1 (CYCLE)"=w186, "1 (T-RISE min)"=w185) -> (w192:T5)
                    n133 = local write "LAB04 (DISP)"(w192) -> ()
                  }
                  frame #7 {
                    # "update cycle value"
                    # "LAB04-2"
                    n134 = local read "LAB04 (DISP)"() -> (w203:T5)
                    n135 = Unbundle By Name(w203) -> ("2 (CYCLE)"=w202:dbl)
                    n136 = case shown="True" w205 {
                      tunnel: [w206 w208] -> w198
                      tunnel: w202 -> [w206 w207]
                      frame False {
                      }
                      frame True {
                        n137 = Increment(x=w207) -> (x+1=w208:dbl)
                      }
                    }
                    n138 = Multiply(x=w198, y=w199) -> (x*y=w201:dbl)
                    n139 = Divide(x=w201, y=60.0) -> (x/y=w197:dbl)
                    n140 = Bundle By Name(cluster=w203, "2 (CYCLE)"=w198, "2 (T-RISE min)"=w197) -> (w204:T5)
                    n141 = local write "LAB04 (DISP)"(w204) -> ()
                  }
                  frame #8 {
                    # "update cycle value"
                    # "LAB05-1"
                    n142 = local read "LAB05 (DISP)"() -> (w215:T5)
                    n143 = Unbundle By Name(w215) -> ("1 (CYCLE)"=w214:dbl)
                    n144 = case shown="True" w217 {
                      tunnel: [w218 w220] -> w210
                      tunnel: w214 -> [w218 w219]
                      frame False {
                      }
                      frame True {
                        n145 = Increment(x=w219) -> (x+1=w220:dbl)
                      }
                    }
                    n146 = Multiply(x=w210, y=w211) -> (x*y=w212:dbl)
                    n147 = Divide(x=w212, y=60.0) -> (x/y=w209:dbl)
                    n148 = Bundle By Name(cluster=w215, "1 (CYCLE)"=w210, "1 (T-RISE min)"=w209) -> (w216:T5)
                    n149 = local write "LAB05 (DISP)"(w216) -> ()
                  }
                  frame #9 {
                    # "update cycle value"
                    # "LAB05-2"
                    n150 = local read "LAB05 (DISP)"() -> (w227:T5)
                    n151 = Unbundle By Name(w227) -> ("2 (CYCLE)"=w226:dbl)
                    n152 = case shown="True" w229 {
                      tunnel: [w230 w232] -> w222
                      tunnel: w226 -> [w230 w231]
                      frame False {
                      }
                      frame True {
                        n153 = Increment(x=w231) -> (x+1=w232:dbl)
                      }
                    }
                    n154 = Multiply(x=w222, y=w223) -> (x*y=w224:dbl)
                    n155 = Divide(x=w224, y=60.0) -> (x/y=w221:dbl)
                    n156 = Bundle By Name(cluster=w227, "2 (CYCLE)"=w222, "2 (T-RISE min)"=w221) -> (w228:T5)
                    n157 = local write "LAB05 (DISP)"(w228) -> ()
                  }
                }
                n158 = local write "jig cycle"(0) -> ()
              }
            }
          }
          frame #3 {
            # "check for RUN switch change, start test if true and stop test if false"
            n159 = Get Date/Time In Seconds() -> (seconds since 1Jan1904=w255:timestamp)
            n160 = Format Date/Time String(time format string (%c)="%Y%m%d", seconds (now)=w255) -> (date/time string=w256:string)  [unwired: 1 in]
            n161 = Format Date/Time String(time format string (%c)="%H%M", seconds (now)=w255) -> (date/time string=w253:string)  [unwired: 1 in]
            n162 = event shown="[9] \"LAB05-1 RUN\": Value Change" {
              selector: _ -> [_ _ _ _ _ _ _ _ _ _ _]
              dyn-events: _ -> [_ _ _ _ _ _ _ _ _ _ _]
              timeout: 10 -> [_ _ _ _ _ _ _ _ _ _ _]
              tunnel: "c:\\crabtree\\Test Data\\" -> [_ w264 w342 w420 w498 w576 w654 w732 w810 w888 w966]
              tunnel: w256 -> [_ w263 w341 w419 w497 w575 w653 w731 w809 w887 w965]
              tunnel: w253 -> [_ w261 w340 w418 w496 w574 w652 w730 w808 w886 w964]
              tunnel: w251 -> [_ w262 _ _ _ _ _ _ _ _ _]
              tunnel: w252 -> [_ w260 _ _ _ _ _ _ _ _ _]
              tunnel: w250 -> [_ _ w339 _ _ _ _ _ _ _ _]
              tunnel: w249 -> [_ _ w338 _ _ _ _ _ _ _ _]
              tunnel: w248 -> [_ _ _ w417 _ _ _ _ _ _ _]
              tunnel: w247 -> [_ _ _ w416 _ _ _ _ _ _ _]
              tunnel: w246 -> [_ _ _ _ w495 _ _ _ _ _ _]
              tunnel: w245 -> [_ _ _ _ w494 _ _ _ _ _ _]
              tunnel: w244 -> [_ _ _ _ _ w573 _ _ _ _ _]
              tunnel: w243 -> [_ _ _ _ _ w572 _ _ _ _ _]
              tunnel: w242 -> [_ _ _ _ _ _ w651 _ _ _ _]
              tunnel: w241 -> [_ _ _ _ _ _ w650 _ _ _ _]
              tunnel: w240 -> [_ _ _ _ _ _ _ w729 _ _ _]
              tunnel: w239 -> [_ _ _ _ _ _ _ w728 _ _ _]
              tunnel: w238 -> [_ _ _ _ _ _ _ _ w807 _ _]
              tunnel: w237 -> [_ _ _ _ _ _ _ _ w806 _ _]
              tunnel: w236 -> [_ _ _ _ _ _ _ _ _ w885 _]
              tunnel: w235 -> [_ _ _ _ _ _ _ _ _ w884 _]
              tunnel: w234 -> [_ _ _ _ _ _ _ _ _ _ w963]
              tunnel: w233 -> [_ _ _ _ _ _ _ _ _ _ w962]
              event Timeout {
                n163 = event-data() -> ()  [unwired: 1 in, 3 out]
              }
              event "LAB01-1RUN": Value Change {
                n164 = event-data() -> ()  [unwired: 1 in, 6 out]
                n165 = case shown="True" w260 {
                  tunnel: w264 -> [_ w286]
                  tunnel: w263 -> [_ w285]
                  tunnel: w262 -> [w265 w284]
                  tunnel: w261 -> [_ w283]
                  frame False {
                    # "stop test"
                    n166 = stacked-sequence {
                      tunnel: w265 -> [w271 _]
                      frame #0 {
                        n167 = local read "LAB01 (DISP)"() -> (w270:T5)
                        n168 = Unbundle(w270) -> ("1 (CYCLE)"=w268:dbl, "1 (T-RISE min)"=w269:dbl)  [unwired: 4 out]
                        n169 = case shown="\"CYCLE TEST\"" w271 {
                          tunnel: w269 -> [_ _ w278]
                          tunnel: w268 -> [w276 w277 _]
                          tunnel: [w276 w277 w278] -> w267
                          frame "TEST SET UP", Default {
                          }
                          frame "CYCLE TEST" {
                          }
                          frame "T-RISE TEST" {
                          }
                        }
                        n170 = local read "LAB01-1 (TDMS)"() -> (w275:refnum<k34>)
                        n171 = Build Array("STOPPED") -> (w272:string[])
                        n172 = Build Array(w267) -> (w266:dbl[])
                        n173 = TDMS Write(0:w275, 5:"TEST RESULT", 7:w272, 9:w266) -> ()  [unwired: 2 in, 4 out]
                      }
                      frame #1 {
                        n174 = local read "LAB01 (DISP)"() -> (w282:T5)
                        n175 = Bundle(cluster=w282, "1 (STATUS)"="STOP") -> (w280:T5)  [unwired: 5 in]
                        n176 = local write "LAB01-1 (RESULT)"(FALSE) -> ()
                        n177 = local write "LAB01 (DISP)"(w280) -> ()
                      }
                    }
                  }
                  frame True {
                    # "start new test and create test file"
                    n178 = stacked-sequence {
                      seq-local: [w292 _ _ _ _] -> [_ w311 _ _ _]
                      tunnel: w286 -> [w301 _ _ _ _]
                      tunnel: w285 -> [w299 _ _ _ _]
                      tunnel: w284 -> [w298 _ _ _ _]
                      tunnel: w283 -> [w289 _ _ _ _]
                      frame #0 {
                        n179 = local read "LAB01 (SET)"() -> (w291:T4)
                        n180 = case shown="\"TEST SET UP\", Default" w298 {
                          tunnel: ["TEST SET UP-" "CYCLE TEST-" "T-RISE TEST-"] -> w294
                          frame "TEST SET UP", Default {
                          }
                          frame "CYCLE TEST" {
                          }
                          frame "T-RISE TEST" {
                          }
                        }
                        n181 = Unbundle(w291) -> ("1 Description"=w290:string)  [unwired: 9 out]
                        n182 = Concatenate Strings(w301, "LAB01-1\\", w299, "\\") -> (w295:string)
                        n183 = String To Path(string=w295) -> (path=w297:path)
                        n184 = Concatenate Strings(w295, w294, w290, "-", w289, ".tdms") -> (w292:string)
                        n185 = Create Folder(path (use dialog)=w297) -> (error out=w296:errorcluster)  [unwired: 2 in, 2 out]
                        n186 = call <vilib>:"Clear Errors.vi"("error in (no error)"=w296) -> ()  [unwired: 6 in, 1 out]
                      }
                      frame #1 {
                        n187 = String To Path(string=w311) -> (path=w305:path)
                        n188 = TDMS Open(5:FALSE, 6:FALSE, 10:T14."create or replace" ("operation (0:open)"), 11:w305) -> (0:w307:errorcluster, 3:→"LAB01-1 (TDMS)":refnum<k34>)  [unwired: 3 in]
                        n189 = local write "data file error"(w307) -> ()
                      }
                      frame #2 {
                        n190 = local read "LAB01 (SET)"() -> (w317:T4)
                        n191 = local read "LAB01-1 (TDMS)"() -> (w328:refnum<k34>)
                        n192 = Build Array("Testers Name", "Description", "Set Test Cycles", "T-Rise minutes", "T-Rise Deg C") -> (w318:string[])
                        n193 = Unbundle(w317) -> ("1 Name"=w316:string, "1 Description"=w315:string, "1 (CYCLES)"=w314:dbl, "1 (T-RISE mins)"=w313:dbl, "1 (T-RISE deg C)"=w312:dbl)  [unwired: 5 out]
                        n194 = Number To Decimal String(number=w314) -> (decimal integer string=w327:string)  [unwired: 1 in]
                        n195 = Number To Decimal String(number=w313) -> (decimal integer string=w326:string)  [unwired: 1 in]
                        n196 = Number To Decimal String(number=w312) -> (decimal integer string=w325:string)  [unwired: 1 in]
                        n197 = Build Array(w316, w315, w327, w326, w325) -> (w324:string[])
                        n198 = TDMS Set Properties(5:w324, 7:w318, 11:w328) -> ()  [unwired: 3 in, 4 out]
                      }
                      frame #3 {
                        w330 = 0.0
                        n199 = local read "LAB01 (DISP)"() -> (w332:T5)
                        n200 = Bundle(cluster=w332, "1 (CYCLE)"=w330, "1 (T-RISE min)"=w330, "1 (STATUS)"="RUN") -> (w331:T5)  [unwired: 3 in]
                        n201 = local write "LAB01 (DISP)"(w331) -> ()
                      }
                      frame #4 {
                        n202 = local read "LAB01-1 (SIG)"() -> (w335:T2)
                        n203 = local read "LAB01 (TEMP START)"() -> (w337:T6)
                        n204 = Unbundle(w335) -> ("Tmp Live"=w334:dbl, "Tmp Neut"=w333:dbl)  [unwired: 3 out]
                        n205 = Bundle(cluster=w337, "1 (TL)"=w334, "1 (TN)"=w333) -> (w336:T6)  [unwired: 2 in]
                        n206 = local write "LAB01 (TEMP START)"(w336) -> ()
                      }
                    }
                  }
                }
              }
              event "LAB01-2 RUN": Value Change {
                n207 = event-data() -> ()  [unwired: 1 in, 6 out]
                n208 = case shown="True" w339 {
                  tunnel: w342 -> [_ w364]
                  tunnel: w341 -> [_ w363]
                  tunnel: w338 -> [w343 w362]
                  tunnel: w340 -> [_ w361]
                  frame False {
                    # "stop test"
                    n209 = stacked-sequence {
                      tunnel: w343 -> [w349 _]
                      frame #0 {
                        n210 = local read "LAB01 (DISP)"() -> (w348:T5)
                        n211 = Unbundle(w348) -> ("2 (CYCLE)"=w344:dbl, "2 (T-RISE min)"=w345:dbl)  [unwired: 4 out]
                        n212 = case shown="\"CYCLE TEST\"" w349 {
                          tunnel: w345 -> [_ _ w356]
                          tunnel: w344 -> [w354 w355 _]
                          tunnel: [w354 w355 w356] -> w347
                          frame "TEST SET UP", Default {
                          }
                          frame "CYCLE TEST" {
                          }
                          frame "T-RISE TEST" {
                          }
                        }
                        n213 = local read "LAB01-2 (TDMS)"() -> (w353:refnum<k34>)
                        n214 = Build Array("STOPPED") -> (w350:string[])
                        n215 = Build Array(w347) -> (w346:dbl[])
                        n216 = TDMS Write(0:w353, 5:"TEST RESULT", 7:w350, 9:w346) -> ()  [unwired: 2 in, 4 out]
                      }
                      frame #1 {
                        n217 = local read "LAB01 (DISP)"() -> (w360:T5)
                        n218 = Bundle(cluster=w360, "2 (STATUS)"="STOP") -> (w359:T5)  [unwired: 5 in]
                        n219 = local write "LAB01-2 (RESULT)"(FALSE) -> ()
                        n220 = local write "LAB01 (DISP)"(w359) -> ()
                      }
                    }
                  }
                  frame True {
                    # "start new test and create test file"
                    n221 = stacked-sequence {
                      seq-local: [w370 _ _ _ _] -> [_ w389 _ _ _]
                      tunnel: w364 -> [w379 _ _ _ _]
                      tunnel: w363 -> [w377 _ _ _ _]
                      tunnel: w362 -> [w376 _ _ _ _]
                      tunnel: w361 -> [w368 _ _ _ _]
                      frame #0 {
                        n222 = local read "LAB01 (SET)"() -> (w369:T4)
                        n223 = case shown="\"TEST SET UP\", Default" w376 {
                          tunnel: ["TEST SET UP-" "CYCLE TEST-" "T-RISE TEST-"] -> w372
                          frame "TEST SET UP", Default {
                          }
                          frame "CYCLE TEST" {
                          }
                          frame "T-RISE TEST" {
                          }
                        }
                        n224 = Unbundle(w369) -> ("2 Description"=w365:string)  [unwired: 9 out]
                        n225 = Concatenate Strings(w379, "LAB01-2\\", w377, "\\") -> (w373:string)
                        n226 = String To Path(string=w373) -> (path=w375:path)
                        n227 = Concatenate Strings(w373, w372, w365, "-", w368, ".tdms") -> (w370:string)
                        n228 = Create Folder(path (use dialog)=w375) -> (error out=w374:errorcluster)  [unwired: 2 in, 2 out]
                        n229 = call <vilib>:"Clear Errors.vi"("error in (no error)"=w374) -> ()  [unwired: 6 in, 1 out]
                      }
                      frame #1 {
                        n230 = String To Path(string=w389) -> (path=w383:path)
                        n231 = TDMS Open(5:FALSE, 6:FALSE, 10:T14."create or replace" ("operation (0:open)"), 11:w383) -> (0:w385:errorcluster, 3:→"LAB01-2 (TDMS)":refnum<k34>)  [unwired: 3 in]
                        n232 = local write "data file error"(w385) -> ()
                      }
                      frame #2 {
                        n233 = local read "LAB01 (SET)"() -> (w395:T4)
                        n234 = local read "LAB01-2 (TDMS)"() -> (w406:refnum<k34>)
                        n235 = Build Array("Testers Name", "Description", "Set Test Cycles", "T-Rise minutes", "T-Rise Deg C") -> (w396:string[])
                        n236 = Unbundle(w395) -> ("2 Name"=w394:string, "2 Description"=w393:string, "2 (CYCLES)"=w392:dbl, "2 (T-RISE mins)"=w391:dbl, "2 (T-RISE deg C)"=w390:dbl)  [unwired: 5 out]
                        n237 = Number To Decimal String(number=w392) -> (decimal integer string=w405:string)  [unwired: 1 in]
                        n238 = Number To Decimal String(number=w391) -> (decimal integer string=w404:string)  [unwired: 1 in]
                        n239 = Number To Decimal String(number=w390) -> (decimal integer string=w403:string)  [unwired: 1 in]
                        n240 = Build Array(w394, w393, w405, w404, w403) -> (w402:string[])
                        n241 = TDMS Set Properties(5:w402, 7:w396, 11:w406) -> ()  [unwired: 3 in, 4 out]
                      }
                      frame #3 {
                        w408 = 0.0
                        n242 = local read "LAB01 (DISP)"() -> (w410:T5)
                        n243 = Bundle(cluster=w410, "2 (CYCLE)"=w408, "2 (T-RISE min)"=w408, "2 (STATUS)"="RUN") -> (w409:T5)  [unwired: 3 in]
                        n244 = local write "LAB01 (DISP)"(w409) -> ()
                      }
                      frame #4 {
                        n245 = local read "LAB01-2 (SIG)"() -> (w413:T2)
                        n246 = local read "LAB01 (TEMP START)"() -> (w415:T6)
                        n247 = Unbundle(w413) -> ("Tmp Live"=w411:dbl, "Tmp Neut"=w412:dbl)  [unwired: 3 out]
                        n248 = Bundle(cluster=w415, "2 (TL)"=w411, "2 (TN)"=w412) -> (w414:T6)  [unwired: 2 in]
                        n249 = local write "LAB01 (TEMP START)"(w414) -> ()
                      }
                    }
                  }
                }
              }
              event "LAB02-1 RUN": Value Change {
                n250 = event-data() -> ()  [unwired: 1 in, 6 out]
                n251 = case shown="True" w417 {
                  tunnel: w420 -> [_ w442]
                  tunnel: w419 -> [_ w441]
                  tunnel: w416 -> [w421 w440]
                  tunnel: w418 -> [_ w439]
                  frame False {
                    # "stop test"
                    n252 = stacked-sequence {
                      tunnel: w421 -> [w427 _]
                      frame #0 {
                        n253 = local read "LAB02 (DISP)"() -> (w426:T5)
                        n254 = Unbundle(w426) -> ("2 (CYCLE)"=w422:dbl, "2 (T-RISE min)"=w423:dbl)  [unwired: 4 out]
                        n255 = case shown="\"CYCLE TEST\"" w427 {
                          tunnel: w423 -> [_ _ w434]
                          tunnel: w422 -> [w432 w433 _]
                          tunnel: [w432 w433 w434] -> w425
                          frame "TEST SET UP", Default {
                          }
                          frame "CYCLE TEST" {
                          }
                          frame "T-RISE TEST" {
                          }
                        }
                        n256 = local read "LAB02-1 (TDMS)"() -> (w431:refnum<k34>)
                        n257 = Build Array("STOPPED") -> (w428:string[])
                        n258 = Build Array(w425) -> (w424:dbl[])
                        n259 = TDMS Write(0:w431, 5:"TEST RESULT", 7:w428, 9:w424) -> ()  [unwired: 2 in, 4 out]
                      }
                      frame #1 {
                        n260 = local read "LAB02 (DISP)"() -> (w438:T5)
                        n261 = Bundle(cluster=w438, "1 (STATUS)"="STOP") -> (w437:T5)  [unwired: 5 in]
                        n262 = local write "LAB02-1 (RESULT)"(FALSE) -> ()
                        n263 = local write "LAB02 (DISP)"(w437) -> ()
                      }
                    }
                  }
                  frame True {
                    # "start new test and create test file"
                    n264 = stacked-sequence {
                      seq-local: [w448 _ _ _ _] -> [_ w467 _ _ _]
                      tunnel: w442 -> [w457 _ _ _ _]
                      tunnel: w441 -> [w455 _ _ _ _]
                      tunnel: w440 -> [w454 _ _ _ _]
                      tunnel: w439 -> [w446 _ _ _ _]
                      frame #0 {
                        n265 = local read "LAB02 (SET)"() -> (w447:T4)
                        n266 = case shown="\"TEST SET UP\", Default" w454 {
                          tunnel: ["TEST SET UP-" "CYCLE TEST-" "T-RISE TEST-"] -> w450
                          frame "TEST SET UP", Default {
                          }
                          frame "CYCLE TEST" {
                          }
                          frame "T-RISE TEST" {
                          }
                        }
                        n267 = Unbundle(w447) -> ("1 Description"=w443:string)  [unwired: 9 out]
                        n268 = Concatenate Strings(w457, "LAB02-1\\", w455, "\\") -> (w451:string)
                        n269 = String To Path(string=w451) -> (path=w453:path)
                        n270 = Concatenate Strings(w451, w450, w443, "-", w446, ".tdms") -> (w448:string)
                        n271 = Create Folder(path (use dialog)=w453) -> (error out=w452:errorcluster)  [unwired: 2 in, 2 out]
                        n272 = call <vilib>:"Clear Errors.vi"("error in (no error)"=w452) -> ()  [unwired: 6 in, 1 out]
                      }
                      frame #1 {
                        n273 = String To Path(string=w467) -> (path=w461:path)
                        n274 = TDMS Open(5:FALSE, 6:FALSE, 10:T14."create or replace" ("operation (0:open)"), 11:w461) -> (0:w463:errorcluster, 3:→"LAB02-1 (TDMS)":refnum<k34>)  [unwired: 3 in]
                        n275 = local write "data file error"(w463) -> ()
                      }
                      frame #2 {
                        n276 = local read "LAB02 (SET)"() -> (w473:T4)
                        n277 = local read "LAB02-1 (TDMS)"() -> (w484:refnum<k34>)
                        n278 = Build Array("Testers Name", "Description", "Set Test Cycles", "T-Rise minutes", "T-Rise Deg C") -> (w474:string[])
                        n279 = Unbundle(w473) -> ("1 Name"=w472:string, "1 Description"=w471:string, "1 (CYCLES)"=w470:dbl, "1 (T-RISE mins)"=w469:dbl, "1 (T-RISE deg C)"=w468:dbl)  [unwired: 5 out]
                        n280 = Number To Decimal String(number=w470) -> (decimal integer string=w483:string)  [unwired: 1 in]
                        n281 = Number To Decimal String(number=w469) -> (decimal integer string=w482:string)  [unwired: 1 in]
                        n282 = Number To Decimal String(number=w468) -> (decimal integer string=w481:string)  [unwired: 1 in]
                        n283 = Build Array(w472, w471, w483, w482, w481) -> (w480:string[])
                        n284 = TDMS Set Properties(5:w480, 7:w474, 11:w484) -> ()  [unwired: 3 in, 4 out]
                      }
                      frame #3 {
                        w486 = 0.0
                        n285 = local read "LAB02 (DISP)"() -> (w488:T5)
                        n286 = Bundle(cluster=w488, "1 (CYCLE)"=w486, "1 (T-RISE min)"=w486, "1 (STATUS)"="RUN") -> (w487:T5)  [unwired: 3 in]
                        n287 = local write "LAB02 (DISP)"(w487) -> ()
                      }
                      frame #4 {
                        n288 = local read "LAB02-1 (SIG)"() -> (w491:T2)
                        n289 = local read "LAB02 (TEMP START)"() -> (w493:T6)
                        n290 = Unbundle(w491) -> ("Tmp Live"=w490:dbl, "Tmp Neut"=w489:dbl)  [unwired: 3 out]
                        n291 = Bundle(cluster=w493, "1 (TL)"=w490, "1 (TN)"=w489) -> (w492:T6)  [unwired: 2 in]
                        n292 = local write "LAB02 (TEMP START)"(w492) -> ()
                      }
                    }
                  }
                }
              }
              event "LAB02-2 RUN": Value Change {
                n293 = event-data() -> ()  [unwired: 1 in, 6 out]
                n294 = case shown="False" w495 {
                  tunnel: w498 -> [_ w520]
                  tunnel: w497 -> [_ w519]
                  tunnel: w494 -> [w499 w518]
                  tunnel: w496 -> [_ w517]
                  frame False {
                    # "stop test"
                    n295 = stacked-sequence {
                      tunnel: w499 -> [w505 _]
                      frame #0 {
                        n296 = local read "LAB02 (DISP)"() -> (w504:T5)
                        n297 = Unbundle(w504) -> ("2 (CYCLE)"=w500:dbl, "2 (T-RISE min)"=w501:dbl)  [unwired: 4 out]
                        n298 = case shown="\"CYCLE TEST\"" w505 {
                          tunnel: w501 -> [_ _ w512]
                          tunnel: w500 -> [w510 w511 _]
                          tunnel: [w510 w511 w512] -> w503
                          frame "TEST SET UP", Default {
                          }
                          frame "CYCLE TEST" {
                          }
                          frame "T-RISE TEST" {
                          }
                        }
                        n299 = local read "LAB02-2 (TDMS)"() -> (w509:refnum<k34>)
                        n300 = Build Array("STOPPED") -> (w506:string[])
                        n301 = Build Array(w503) -> (w502:dbl[])
                        n302 = TDMS Write(0:w509, 5:"TEST RESULT", 7:w506, 9:w502) -> ()  [unwired: 2 in, 4 out]
                      }
                      frame #1 {
                        n303 = local read "LAB02 (DISP)"() -> (w516:T5)
                        n304 = Bundle(cluster=w516, "2 (STATUS)"="STOP") -> (w515:T5)  [unwired: 5 in]
                        n305 = local write "LAB02-2 (RESULT)"(FALSE) -> ()
                        n306 = local write "LAB02 (DISP)"(w515) -> ()
                      }
                    }
                  }
                  frame True {
                    # "start new test and create test file"
                    n307 = stacked-sequence {
                      seq-local: [w526 _ _ _ _] -> [_ w545 _ _ _]
                      tunnel: w520 -> [w535 _ _ _ _]
                      tunnel: w519 -> [w533 _ _ _ _]
                      tunnel: w518 -> [w532 _ _ _ _]
                      tunnel: w517 -> [w524 _ _ _ _]
                      frame #0 {
                        n308 = local read "LAB02 (SET)"() -> (w525:T4)
                        n309 = case shown="\"TEST SET UP\", Default" w532 {
                          tunnel: ["TEST SET UP-" "CYCLE TEST-" "T-RISE TEST-"] -> w528
                          frame "TEST SET UP", Default {
                          }
                          frame "CYCLE TEST" {
                          }
                          frame "T-RISE TEST" {
                          }
                        }
                        n310 = Unbundle(w525) -> ("2 Description"=w521:string)  [unwired: 9 out]
                        n311 = Concatenate Strings(w535, "LAB02-2\\", w533, "\\") -> (w529:string)
                        n312 = String To Path(string=w529) -> (path=w531:path)
                        n313 = Concatenate Strings(w529, w528, w521, "-", w524, ".tdms") -> (w526:string)
                        n314 = Create Folder(path (use dialog)=w531) -> (error out=w530:errorcluster)  [unwired: 2 in, 2 out]
                        n315 = call <vilib>:"Clear Errors.vi"("error in (no error)"=w530) -> ()  [unwired: 6 in, 1 out]
                      }
                      frame #1 {
                        n316 = String To Path(string=w545) -> (path=w539:path)
                        n317 = TDMS Open(5:FALSE, 6:FALSE, 10:T14."create or replace" ("operation (0:open)"), 11:w539) -> (0:w541:errorcluster, 3:→"LAB02-2 (TDMS)":refnum<k34>)  [unwired: 3 in]
                        n318 = local write "data file error"(w541) -> ()
                      }
                      frame #2 {
                        n319 = local read "LAB02 (SET)"() -> (w551:T4)
                        n320 = local read "LAB02-2 (TDMS)"() -> (w562:refnum<k34>)
                        n321 = Build Array("Testers Name", "Description", "Set Test Cycles", "T-Rise minutes", "T-Rise Deg C") -> (w552:string[])
                        n322 = Unbundle(w551) -> ("2 Name"=w546:string, "2 Description"=w547:string, "2 (CYCLES)"=w548:dbl, "2 (T-RISE mins)"=w549:dbl, "2 (T-RISE deg C)"=w550:dbl)  [unwired: 5 out]
                        n323 = Number To Decimal String(number=w548) -> (decimal integer string=w561:string)  [unwired: 1 in]
                        n324 = Number To Decimal String(number=w549) -> (decimal integer string=w560:string)  [unwired: 1 in]
                        n325 = Number To Decimal String(number=w550) -> (decimal integer string=w559:string)  [unwired: 1 in]
                        n326 = Build Array(w546, w547, w561, w560, w559) -> (w558:string[])
                        n327 = TDMS Set Properties(5:w558, 7:w552, 11:w562) -> ()  [unwired: 3 in, 4 out]
                      }
                      frame #3 {
                        w563 = 0.0
                        n328 = local read "LAB02 (DISP)"() -> (w566:T5)
                        n329 = Bundle(cluster=w566, "2 (CYCLE)"=w563, "2 (T-RISE min)"=w563, "2 (STATUS)"="RUN") -> (w565:T5)  [unwired: 3 in]
                        n330 = local write "LAB02 (DISP)"(w565) -> ()
                      }
                      frame #4 {
                        n331 = local read "LAB02-2 (SIG)"() -> (w569:T2)
                        n332 = local read "LAB02 (TEMP START)"() -> (w571:T6)
                        n333 = Unbundle(w569) -> ("Tmp Live"=w567:dbl, "Tmp Neut"=w568:dbl)  [unwired: 3 out]
                        n334 = Bundle(cluster=w571, "2 (TL)"=w567, "2 (TN)"=w568) -> (w570:T6)  [unwired: 2 in]
                        n335 = local write "LAB02 (TEMP START)"(w570) -> ()
                      }
                    }
                  }
                }
              }
              event "LAB03-1 RUN": Value Change {
                n336 = event-data() -> ()  [unwired: 1 in, 6 out]
                n337 = case shown="True" w573 {
                  tunnel: w576 -> [_ w598]
                  tunnel: w575 -> [_ w597]
                  tunnel: w572 -> [w577 w596]
                  tunnel: w574 -> [_ w595]
                  frame False {
                    # "stop test"
                    n338 = stacked-sequence {
                      tunnel: w577 -> [w583 _]
                      frame #0 {
                        n339 = local read "LAB03 (DISP)"() -> (w582:T5)
                        n340 = Unbundle(w582) -> ("1 (CYCLE)"=w579:dbl, "1 (T-RISE min)"=w578:dbl)  [unwired: 4 out]
                        n341 = case shown="\"CYCLE TEST\"" w583 {
                          tunnel: w578 -> [_ _ w590]
                          tunnel: w579 -> [w588 w589 _]
                          tunnel: [w588 w589 w590] -> w581
                          frame "TEST SET UP", Default {
                          }
                          frame "CYCLE TEST" {
                          }
                          frame "T-RISE TEST" {
                          }
                        }
                        n342 = local read "LAB03-1 (TDMS)"() -> (w587:refnum<k34>)
                        n343 = Build Array("STOPPED") -> (w584:string[])
                        n344 = Build Array(w581) -> (w580:dbl[])
                        n345 = TDMS Write(0:w587, 5:"TEST RESULT", 7:w584, 9:w580) -> ()  [unwired: 2 in, 4 out]
                      }
                      frame #1 {
                        n346 = local read "LAB03 (DISP)"() -> (w594:T5)
                        n347 = Bundle(cluster=w594, "1 (STATUS)"="STOP") -> (w593:T5)  [unwired: 5 in]
                        n348 = local write "LAB03-1 (RESULT)"(FALSE) -> ()
                        n349 = local write "LAB03 (DISP)"(w593) -> ()
                      }
                    }
                  }
                  frame True {
                    # "start new test and create test file"
                    n350 = stacked-sequence {
                      seq-local: [w604 _ _ _ _] -> [_ w623 _ _ _]
                      tunnel: w598 -> [w613 _ _ _ _]
                      tunnel: w597 -> [w611 _ _ _ _]
                      tunnel: w596 -> [w610 _ _ _ _]
                      tunnel: w595 -> [w602 _ _ _ _]
                      frame #0 {
                        n351 = local read "LAB03 (SET)"() -> (w603:T4)
                        n352 = case shown="\"TEST SET UP\", Default" w610 {
                          tunnel: ["TEST SET UP-" "CYCLE TEST-" "T-RISE TEST-"] -> w606
                          frame "TEST SET UP", Default {
                          }
                          frame "CYCLE TEST" {
                          }
                          frame "T-RISE TEST" {
                          }
                        }
                        n353 = Unbundle(w603) -> ("1 Description"=w599:string)  [unwired: 9 out]
                        n354 = Concatenate Strings(w613, "LAB03-1\\", w611, "\\") -> (w607:string)
                        n355 = String To Path(string=w607) -> (path=w609:path)
                        n356 = Concatenate Strings(w607, w606, w599, "-", w602, ".tdms") -> (w604:string)
                        n357 = Create Folder(path (use dialog)=w609) -> (error out=w608:errorcluster)  [unwired: 2 in, 2 out]
                        n358 = call <vilib>:"Clear Errors.vi"("error in (no error)"=w608) -> ()  [unwired: 6 in, 1 out]
                      }
                      frame #1 {
                        n359 = String To Path(string=w623) -> (path=w617:path)
                        n360 = TDMS Open(5:FALSE, 6:FALSE, 10:T14."create or replace" ("operation (0:open)"), 11:w617) -> (0:w619:errorcluster, 3:→"LAB03-1 (TDMS)":refnum<k34>)  [unwired: 3 in]
                        n361 = local write "data file error"(w619) -> ()
                      }
                      frame #2 {
                        n362 = local read "LAB03 (SET)"() -> (w629:T4)
                        n363 = local read "LAB03-1 (TDMS)"() -> (w640:refnum<k34>)
                        n364 = Build Array("Testers Name", "Description", "Set Test Cycles", "T-Rise minutes", "T-Rise Deg C") -> (w630:string[])
                        n365 = Unbundle(w629) -> ("1 Name"=w628:string, "1 Description"=w627:string, "1 (CYCLES)"=w626:dbl, "1 (T-RISE mins)"=w625:dbl, "1 (T-RISE deg C)"=w624:dbl)  [unwired: 5 out]
                        n366 = Number To Decimal String(number=w626) -> (decimal integer string=w639:string)  [unwired: 1 in]
                        n367 = Number To Decimal String(number=w625) -> (decimal integer string=w638:string)  [unwired: 1 in]
                        n368 = Number To Decimal String(number=w624) -> (decimal integer string=w637:string)  [unwired: 1 in]
                        n369 = Build Array(w628, w627, w639, w638, w637) -> (w636:string[])
                        n370 = TDMS Set Properties(5:w636, 7:w630, 11:w640) -> ()  [unwired: 3 in, 4 out]
                      }
                      frame #3 {
                        w642 = 0.0
                        n371 = local read "LAB03 (DISP)"() -> (w644:T5)
                        n372 = Bundle(cluster=w644, "1 (CYCLE)"=w642, "1 (T-RISE min)"=w642, "1 (STATUS)"="RUN") -> (w643:T5)  [unwired: 3 in]
                        n373 = local write "LAB03 (DISP)"(w643) -> ()
                      }
                      frame #4 {
                        n374 = local read "LAB03-1 (SIG)"() -> (w647:T2)
                        n375 = local read "LAB03 (TEMP START)"() -> (w649:T6)
                        n376 = Unbundle(w647) -> ("Tmp Live"=w646:dbl, "Tmp Neut"=w645:dbl)  [unwired: 3 out]
                        n377 = Bundle(cluster=w649, "1 (TL)"=w646, "1 (TN)"=w645) -> (w648:T6)  [unwired: 2 in]
                        n378 = local write "LAB03 (TEMP START)"(w648) -> ()
                      }
                    }
                  }
                }
              }
              event "LAB03-2 RUN": Value Change {
                n379 = event-data() -> ()  [unwired: 1 in, 6 out]
                n380 = case shown="True" w651 {
                  tunnel: w654 -> [_ w676]
                  tunnel: w653 -> [_ w675]
                  tunnel: w650 -> [w655 w674]
                  tunnel: w652 -> [_ w673]
                  frame False {
                    # "stop test"
                    n381 = stacked-sequence {
                      tunnel: w655 -> [w661 _]
                      frame #0 {
                        n382 = local read "LAB03 (DISP)"() -> (w660:T5)
                        n383 = Unbundle(w660) -> ("2 (CYCLE)"=w656:dbl, "2 (T-RISE min)"=w657:dbl)  [unwired: 4 out]
                        n384 = case shown="\"CYCLE TEST\"" w661 {
                          tunnel: w657 -> [_ _ w668]
                          tunnel: w656 -> [w666 w667 _]
                          tunnel: [w666 w667 w668] -> w659
                          frame "TEST SET UP", Default {
                          }
                          frame "CYCLE TEST" {
                          }
                          frame "T-RISE TEST" {
                          }
                        }
                        n385 = local read "LAB03-2 (TDMS)"() -> (w665:refnum<k34>)
                        n386 = Build Array("STOPPED") -> (w662:string[])
                        n387 = Build Array(w659) -> (w658:dbl[])
                        n388 = TDMS Write(0:w665, 5:"TEST RESULT", 7:w662, 9:w658) -> ()  [unwired: 2 in, 4 out]
                      }
                      frame #1 {
                        n389 = local read "LAB03 (DISP)"() -> (w672:T5)
                        n390 = Bundle(cluster=w672, "2 (STATUS)"="STOP") -> (w671:T5)  [unwired: 5 in]
                        n391 = local write "LAB03-2 (RESULT)"(FALSE) -> ()
                        n392 = local write "LAB03 (DISP)"(w671) -> ()
                      }
                    }
                  }
                  frame True {
                    # "start new test and create test file"
                    n393 = stacked-sequence {
                      seq-local: [w682 _ _ _ _] -> [_ w701 _ _ _]
                      tunnel: w676 -> [w691 _ _ _ _]
                      tunnel: w675 -> [w689 _ _ _ _]
                      tunnel: w674 -> [w688 _ _ _ _]
                      tunnel: w673 -> [w680 _ _ _ _]
                      frame #0 {
                        n394 = local read "LAB03 (SET)"() -> (w681:T4)
                        n395 = case shown="\"TEST SET UP\", Default" w688 {
                          tunnel: ["TEST SET UP-" "CYCLE TEST-" "T-RISE TEST-"] -> w684
                          frame "TEST SET UP", Default {
                          }
                          frame "CYCLE TEST" {
                          }
                          frame "T-RISE TEST" {
                          }
                        }
                        n396 = Unbundle(w681) -> ("2 Description"=w677:string)  [unwired: 9 out]
                        n397 = Concatenate Strings(w691, "LAB03-2\\", w689, "\\") -> (w685:string)
                        n398 = String To Path(string=w685) -> (path=w687:path)
                        n399 = Concatenate Strings(w685, w684, w677, "-", w680, ".tdms") -> (w682:string)
                        n400 = Create Folder(path (use dialog)=w687) -> (error out=w686:errorcluster)  [unwired: 2 in, 2 out]
                        n401 = call <vilib>:"Clear Errors.vi"("error in (no error)"=w686) -> ()  [unwired: 6 in, 1 out]
                      }
                      frame #1 {
                        n402 = String To Path(string=w701) -> (path=w695:path)
                        n403 = TDMS Open(5:FALSE, 6:FALSE, 10:T14."create or replace" ("operation (0:open)"), 11:w695) -> (0:w697:errorcluster, 3:→"LAB03-2 (TDMS)":refnum<k34>)  [unwired: 3 in]
                        n404 = local write "data file error"(w697) -> ()
                      }
                      frame #2 {
                        n405 = local read "LAB03 (SET)"() -> (w707:T4)
                        n406 = local read "LAB03-2 (TDMS)"() -> (w718:refnum<k34>)
                        n407 = Build Array("Testers Name", "Description", "Set Test Cycles", "T-Rise minutes", "T-Rise Deg C") -> (w708:string[])
                        n408 = Unbundle(w707) -> ("2 Name"=w706:string, "2 Description"=w705:string, "2 (CYCLES)"=w704:dbl, "2 (T-RISE mins)"=w703:dbl, "2 (T-RISE deg C)"=w702:dbl)  [unwired: 5 out]
                        n409 = Number To Decimal String(number=w704) -> (decimal integer string=w717:string)  [unwired: 1 in]
                        n410 = Number To Decimal String(number=w703) -> (decimal integer string=w716:string)  [unwired: 1 in]
                        n411 = Number To Decimal String(number=w702) -> (decimal integer string=w715:string)  [unwired: 1 in]
                        n412 = Build Array(w706, w705, w717, w716, w715) -> (w714:string[])
                        n413 = TDMS Set Properties(5:w714, 7:w708, 11:w718) -> ()  [unwired: 3 in, 4 out]
                      }
                      frame #3 {
                        w720 = 0.0
                        n414 = local read "LAB03 (DISP)"() -> (w722:T5)
                        n415 = Bundle(cluster=w722, "2 (CYCLE)"=w720, "2 (T-RISE min)"=w720, "2 (STATUS)"="RUN") -> (w721:T5)  [unwired: 3 in]
                        n416 = local write "LAB03 (DISP)"(w721) -> ()
                      }
                      frame #4 {
                        n417 = local read "LAB03-2 (SIG)"() -> (w725:T2)
                        n418 = local read "LAB03 (TEMP START)"() -> (w727:T6)
                        n419 = Unbundle(w725) -> ("Tmp Live"=w723:dbl, "Tmp Neut"=w724:dbl)  [unwired: 3 out]
                        n420 = Bundle(cluster=w727, "2 (TL)"=w723, "2 (TN)"=w724) -> (w726:T6)  [unwired: 2 in]
                        n421 = local write "LAB03 (TEMP START)"(w726) -> ()
                      }
                    }
                  }
                }
              }
              event "LAB04-1 RUN": Value Change {
                n422 = event-data() -> ()  [unwired: 1 in, 6 out]
                n423 = case shown="False" w729 {
                  tunnel: w732 -> [_ w754]
                  tunnel: w731 -> [_ w753]
                  tunnel: w728 -> [w733 w752]
                  tunnel: w730 -> [_ w751]
                  frame False {
                    # "stop test"
                    n424 = stacked-sequence {
                      tunnel: w733 -> [w739 _]
                      frame #0 {
                        n425 = local read "LAB04 (DISP)"() -> (w738:T5)
                        n426 = Unbundle(w738) -> ("1 (CYCLE)"=w735:dbl, "1 (T-RISE min)"=w734:dbl)  [unwired: 4 out]
                        n427 = case shown="\"CYCLE TEST\"" w739 {
                          tunnel: w734 -> [_ _ w746]
                          tunnel: w735 -> [w744 w745 _]
                          tunnel: [w744 w745 w746] -> w737
                          frame "TEST SET UP", Default {
                          }
                          frame "CYCLE TEST" {
                          }
                          frame "T-RISE TEST" {
                          }
                        }
                        n428 = local read "LAB04-1 (TDMS)"() -> (w743:refnum<k34>)
                        n429 = Build Array("STOPPED") -> (w740:string[])
                        n430 = Build Array(w737) -> (w736:dbl[])
                        n431 = TDMS Write(0:w743, 5:"TEST RESULT", 7:w740, 9:w736) -> ()  [unwired: 2 in, 4 out]
                      }
                      frame #1 {
                        n432 = local read "LAB04 (DISP)"() -> (w750:T5)
                        n433 = Bundle(cluster=w750, "1 (STATUS)"="STOP") -> (w749:T5)  [unwired: 5 in]
                        n434 = local write "LAB04-1 (RESULT)"(FALSE) -> ()
                        n435 = local write "LAB04 (DISP)"(w749) -> ()
                      }
                    }
                  }
                  frame True {
                    # "start new test and create test file"
                    n436 = stacked-sequence {
                      seq-local: [w760 _ _ _ _] -> [_ w779 _ _ _]
                      tunnel: w754 -> [w769 _ _ _ _]
                      tunnel: w753 -> [w767 _ _ _ _]
                      tunnel: w752 -> [w766 _ _ _ _]
                      tunnel: w751 -> [w758 _ _ _ _]
                      frame #0 {
                        n437 = local read "LAB04 (SET)"() -> (w759:T4)
                        n438 = case shown="\"TEST SET UP\", Default" w766 {
                          tunnel: ["TEST SET UP-" "CYCLE TEST-" "T-RISE TEST-"] -> w762
                          frame "TEST SET UP", Default {
                          }
                          frame "CYCLE TEST" {
                          }
                          frame "T-RISE TEST" {
                          }
                        }
                        n439 = Unbundle(w759) -> ("1 Description"=w755:string)  [unwired: 9 out]
                        n440 = Concatenate Strings(w769, "LAB04-1\\", w767, "\\") -> (w763:string)
                        n441 = String To Path(string=w763) -> (path=w765:path)
                        n442 = Concatenate Strings(w763, w762, w755, "-", w758, ".tdms") -> (w760:string)
                        n443 = Create Folder(path (use dialog)=w765) -> (error out=w764:errorcluster)  [unwired: 2 in, 2 out]
                        n444 = call <vilib>:"Clear Errors.vi"("error in (no error)"=w764) -> ()  [unwired: 6 in, 1 out]
                      }
                      frame #1 {
                        n445 = String To Path(string=w779) -> (path=w773:path)
                        n446 = TDMS Open(5:FALSE, 6:FALSE, 10:T14."create or replace" ("operation (0:open)"), 11:w773) -> (0:w775:errorcluster, 3:→"LAB04-1 (TDMS)":refnum<k34>)  [unwired: 3 in]
                        n447 = local write "data file error"(w775) -> ()
                      }
                      frame #2 {
                        n448 = local read "LAB04 (SET)"() -> (w785:T4)
                        n449 = local read "LAB04-1 (TDMS)"() -> (w796:refnum<k34>)
                        n450 = Build Array("Testers Name", "Description", "Set Test Cycles", "T-Rise minutes", "T-Rise Deg C") -> (w786:string[])
                        n451 = Unbundle(w785) -> ("1 Name"=w784:string, "1 Description"=w783:string, "1 (CYCLES)"=w782:dbl, "1 (T-RISE mins)"=w781:dbl, "1 (T-RISE deg C)"=w780:dbl)  [unwired: 5 out]
                        n452 = Number To Decimal String(number=w782) -> (decimal integer string=w795:string)  [unwired: 1 in]
                        n453 = Number To Decimal String(number=w781) -> (decimal integer string=w794:string)  [unwired: 1 in]
                        n454 = Number To Decimal String(number=w780) -> (decimal integer string=w793:string)  [unwired: 1 in]
                        n455 = Build Array(w784, w783, w795, w794, w793) -> (w792:string[])
                        n456 = TDMS Set Properties(5:w792, 7:w786, 11:w796) -> ()  [unwired: 3 in, 4 out]
                      }
                      frame #3 {
                        w798 = 0.0
                        n457 = local read "LAB04 (DISP)"() -> (w800:T5)
                        n458 = Bundle(cluster=w800, "1 (CYCLE)"=w798, "1 (T-RISE min)"=w798, "1 (STATUS)"="RUN") -> (w799:T5)  [unwired: 3 in]
                        n459 = local write "LAB04 (DISP)"(w799) -> ()
                      }
                      frame #4 {
                        n460 = local read "LAB04-1 (SIG)"() -> (w803:T2)
                        n461 = local read "LAB04 (TEMP START)"() -> (w805:T6)
                        n462 = Unbundle(w803) -> ("Tmp Live"=w802:dbl, "Tmp Neut"=w801:dbl)  [unwired: 3 out]
                        n463 = Bundle(cluster=w805, "1 (TL)"=w802, "1 (TN)"=w801) -> (w804:T6)  [unwired: 2 in]
                        n464 = local write "LAB04 (TEMP START)"(w804) -> ()
                      }
                    }
                  }
                }
              }
              event "LAB04-2 RUN": Value Change {
                n465 = event-data() -> ()  [unwired: 1 in, 6 out]
                n466 = case shown="False" w807 {
                  tunnel: w810 -> [_ w832]
                  tunnel: w809 -> [_ w831]
                  tunnel: w806 -> [w811 w830]
                  tunnel: w808 -> [_ w829]
                  frame False {
                    # "stop test"
                    n467 = stacked-sequence {
                      tunnel: w811 -> [w817 _]
                      frame #0 {
                        n468 = local read "LAB04 (DISP)"() -> (w816:T5)
                        n469 = Unbundle(w816) -> ("2 (CYCLE)"=w813:dbl, "2 (T-RISE min)"=w812:dbl)  [unwired: 4 out]
                        n470 = case shown="\"CYCLE TEST\"" w817 {
                          tunnel: w812 -> [_ _ w824]
                          tunnel: w813 -> [w822 w823 _]
                          tunnel: [w822 w823 w824] -> w815
                          frame "TEST SET UP", Default {
                          }
                          frame "CYCLE TEST" {
                          }
                          frame "T-RISE TEST" {
                          }
                        }
                        n471 = local read "LAB04-2 (TDMS)"() -> (w821:refnum<k34>)
                        n472 = Build Array("STOPPED") -> (w818:string[])
                        n473 = Build Array(w815) -> (w814:dbl[])
                        n474 = TDMS Write(0:w821, 5:"TEST RESULT", 7:w818, 9:w814) -> ()  [unwired: 2 in, 4 out]
                      }
                      frame #1 {
                        n475 = local read "LAB04 (DISP)"() -> (w828:T5)
                        n476 = Bundle(cluster=w828, "2 (STATUS)"="STOP") -> (w827:T5)  [unwired: 5 in]
                        n477 = local write "LAB04-2 (RESULT)"(FALSE) -> ()
                        n478 = local write "LAB04 (DISP)"(w827) -> ()
                      }
                    }
                  }
                  frame True {
                    # "start new test and create test file"
                    n479 = stacked-sequence {
                      seq-local: [w838 _ _ _ _] -> [_ w857 _ _ _]
                      tunnel: w832 -> [w847 _ _ _ _]
                      tunnel: w831 -> [w845 _ _ _ _]
                      tunnel: w830 -> [w844 _ _ _ _]
                      tunnel: w829 -> [w836 _ _ _ _]
                      frame #0 {
                        n480 = local read "LAB04 (SET)"() -> (w837:T4)
                        n481 = case shown="\"TEST SET UP\", Default" w844 {
                          tunnel: ["TEST SET UP-" "CYCLE TEST-" "T-RISE TEST-"] -> w840
                          frame "TEST SET UP", Default {
                          }
                          frame "CYCLE TEST" {
                          }
                          frame "T-RISE TEST" {
                          }
                        }
                        n482 = Unbundle(w837) -> ("2 Description"=w833:string)  [unwired: 9 out]
                        n483 = Concatenate Strings(w847, "LAB04-2\\", w845, "\\") -> (w841:string)
                        n484 = String To Path(string=w841) -> (path=w843:path)
                        n485 = Concatenate Strings(w841, w840, w833, "-", w836, ".tdms") -> (w838:string)
                        n486 = Create Folder(path (use dialog)=w843) -> (error out=w842:errorcluster)  [unwired: 2 in, 2 out]
                        n487 = call <vilib>:"Clear Errors.vi"("error in (no error)"=w842) -> ()  [unwired: 6 in, 1 out]
                      }
                      frame #1 {
                        n488 = String To Path(string=w857) -> (path=w851:path)
                        n489 = TDMS Open(5:FALSE, 6:FALSE, 10:T14."create or replace" ("operation (0:open)"), 11:w851) -> (0:w853:errorcluster, 3:→"LAB04-2 (TDMS)":refnum<k34>)  [unwired: 3 in]
                        n490 = local write "data file error"(w853) -> ()
                      }
                      frame #2 {
                        n491 = local read "LAB04 (SET)"() -> (w863:T4)
                        n492 = local read "LAB04-2 (TDMS)"() -> (w874:refnum<k34>)
                        n493 = Build Array("Testers Name", "Description", "Set Test Cycles", "T-Rise minutes", "T-Rise Deg C") -> (w864:string[])
                        n494 = Unbundle(w863) -> ("2 Name"=w862:string, "2 Description"=w861:string, "2 (CYCLES)"=w860:dbl, "2 (T-RISE mins)"=w859:dbl, "2 (T-RISE deg C)"=w858:dbl)  [unwired: 5 out]
                        n495 = Number To Decimal String(number=w860) -> (decimal integer string=w873:string)  [unwired: 1 in]
                        n496 = Number To Decimal String(number=w859) -> (decimal integer string=w872:string)  [unwired: 1 in]
                        n497 = Number To Decimal String(number=w858) -> (decimal integer string=w871:string)  [unwired: 1 in]
                        n498 = Build Array(w862, w861, w873, w872, w871) -> (w870:string[])
                        n499 = TDMS Set Properties(5:w870, 7:w864, 11:w874) -> ()  [unwired: 3 in, 4 out]
                      }
                      frame #3 {
                        w876 = 0.0
                        n500 = local read "LAB04 (DISP)"() -> (w878:T5)
                        n501 = Bundle(cluster=w878, "2 (CYCLE)"=w876, "2 (T-RISE min)"=w876, "2 (STATUS)"="RUN") -> (w877:T5)  [unwired: 3 in]
                        n502 = local write "LAB04 (DISP)"(w877) -> ()
                      }
                      frame #4 {
                        n503 = local read "LAB04-2 (SIG)"() -> (w881:T2)
                        n504 = local read "LAB04 (TEMP START)"() -> (w883:T6)
                        n505 = Unbundle(w881) -> ("Tmp Live"=w880:dbl, "Tmp Neut"=w879:dbl)  [unwired: 3 out]
                        n506 = Bundle(cluster=w883, "2 (TL)"=w880, "2 (TN)"=w879) -> (w882:T6)  [unwired: 2 in]
                        n507 = local write "LAB04 (TEMP START)"(w882) -> ()
                      }
                    }
                  }
                }
              }
              event "LAB05-1 RUN": Value Change {
                n508 = event-data() -> ()  [unwired: 1 in, 6 out]
                n509 = case shown="False" w885 {
                  tunnel: w888 -> [_ w910]
                  tunnel: w887 -> [_ w909]
                  tunnel: w884 -> [w889 w908]
                  tunnel: w886 -> [_ w907]
                  frame False {
                    # "stop test"
                    n510 = stacked-sequence {
                      tunnel: w889 -> [w895 _]
                      frame #0 {
                        n511 = local read "LAB05 (DISP)"() -> (w894:T5)
                        n512 = Unbundle(w894) -> ("1 (CYCLE)"=w891:dbl, "1 (T-RISE min)"=w890:dbl)  [unwired: 4 out]
                        n513 = case shown="\"CYCLE TEST\"" w895 {
                          tunnel: w890 -> [_ _ w902]
                          tunnel: w891 -> [w900 w901 _]
                          tunnel: [w900 w901 w902] -> w893
                          frame "TEST SET UP", Default {
                          }
                          frame "CYCLE TEST" {
                          }
                          frame "T-RISE TEST" {
                          }
                        }
                        n514 = local read "LAB05-1 (TDMS)"() -> (w899:refnum<k34>)
                        n515 = Build Array("STOPPED") -> (w896:string[])
                        n516 = Build Array(w893) -> (w892:dbl[])
                        n517 = TDMS Write(0:w899, 5:"TEST RESULT", 7:w896, 9:w892) -> ()  [unwired: 2 in, 4 out]
                      }
                      frame #1 {
                        n518 = local read "LAB05 (DISP)"() -> (w906:T5)
                        n519 = Bundle(cluster=w906, "1 (STATUS)"="STOP") -> (w905:T5)  [unwired: 5 in]
                        n520 = local write "LAB05-1 (RESULT)"(FALSE) -> ()
                        n521 = local write "LAB05 (DISP)"(w905) -> ()
                      }
                    }
                  }
                  frame True {
                    # "start new test and create test file"
                    n522 = stacked-sequence {
                      seq-local: [w916 _ _ _ _] -> [_ w935 _ _ _]
                      tunnel: w910 -> [w925 _ _ _ _]
                      tunnel: w909 -> [w923 _ _ _ _]
                      tunnel: w908 -> [w922 _ _ _ _]
                      tunnel: w907 -> [w914 _ _ _ _]
                      frame #0 {
                        n523 = local read "LAB05 (SET)"() -> (w915:T4)
                        n524 = case shown="\"TEST SET UP\", Default" w922 {
                          tunnel: ["TEST SET UP-" "CYCLE TEST-" "T-RISE TEST-"] -> w918
                          frame "TEST SET UP", Default {
                          }
                          frame "CYCLE TEST" {
                          }
                          frame "T-RISE TEST" {
                          }
                        }
                        n525 = Unbundle(w915) -> ("1 Description"=w911:string)  [unwired: 9 out]
                        n526 = Concatenate Strings(w925, "LAB05-1\\", w923, "\\") -> (w919:string)
                        n527 = String To Path(string=w919) -> (path=w921:path)
                        n528 = Concatenate Strings(w919, w918, w911, "-", w914, ".tdms") -> (w916:string)
                        n529 = Create Folder(path (use dialog)=w921) -> (error out=w920:errorcluster)  [unwired: 2 in, 2 out]
                        n530 = call <vilib>:"Clear Errors.vi"("error in (no error)"=w920) -> ()  [unwired: 6 in, 1 out]
                      }
                      frame #1 {
                        n531 = String To Path(string=w935) -> (path=w929:path)
                        n532 = TDMS Open(5:FALSE, 6:FALSE, 10:T14."create or replace" ("operation (0:open)"), 11:w929) -> (0:w931:errorcluster, 3:→"LAB05-1 (TDMS)":refnum<k34>)  [unwired: 3 in]
                        n533 = local write "data file error"(w931) -> ()
                      }
                      frame #2 {
                        n534 = local read "LAB05 (SET)"() -> (w941:T4)
                        n535 = local read "LAB05-1 (TDMS)"() -> (w952:refnum<k34>)
                        n536 = Build Array("Testers Name", "Description", "Set Test Cycles", "T-Rise minutes", "T-Rise Deg C") -> (w942:string[])
                        n537 = Unbundle(w941) -> ("1 Name"=w940:string, "1 Description"=w939:string, "1 (CYCLES)"=w938:dbl, "1 (T-RISE mins)"=w937:dbl, "1 (T-RISE deg C)"=w936:dbl)  [unwired: 5 out]
                        n538 = Number To Decimal String(number=w938) -> (decimal integer string=w951:string)  [unwired: 1 in]
                        n539 = Number To Decimal String(number=w937) -> (decimal integer string=w950:string)  [unwired: 1 in]
                        n540 = Number To Decimal String(number=w936) -> (decimal integer string=w949:string)  [unwired: 1 in]
                        n541 = Build Array(w940, w939, w951, w950, w949) -> (w948:string[])
                        n542 = TDMS Set Properties(5:w948, 7:w942, 11:w952) -> ()  [unwired: 3 in, 4 out]
                      }
                      frame #3 {
                        w954 = 0.0
                        n543 = local read "LAB05 (DISP)"() -> (w956:T5)
                        n544 = Bundle(cluster=w956, "1 (CYCLE)"=w954, "1 (T-RISE min)"=w954, "1 (STATUS)"="RUN") -> (w955:T5)  [unwired: 3 in]
                        n545 = local write "LAB05 (DISP)"(w955) -> ()
                      }
                      frame #4 {
                        n546 = local read "LAB05-1 (SIG)"() -> (w959:T2)
                        n547 = local read "LAB05 (TEMP START)"() -> (w961:T6)
                        n548 = Unbundle(w959) -> ("Tmp Live"=w958:dbl, "Tmp Neut"=w957:dbl)  [unwired: 3 out]
                        n549 = Bundle(cluster=w961, "1 (TL)"=w958, "1 (TN)"=w957) -> (w960:T6)  [unwired: 2 in]
                        n550 = local write "LAB05 (TEMP START)"(w960) -> ()
                      }
                    }
                  }
                }
              }
              event "LAB05-2 RUN": Value Change {
                n551 = event-data() -> ()  [unwired: 1 in, 6 out]
                n552 = case shown="False" w963 {
                  tunnel: w966 -> [_ w988]
                  tunnel: w965 -> [_ w987]
                  tunnel: w962 -> [w967 w986]
                  tunnel: w964 -> [_ w985]
                  frame False {
                    # "stop test"
                    n553 = stacked-sequence {
                      tunnel: w967 -> [w973 _]
                      frame #0 {
                        n554 = local read "LAB05 (DISP)"() -> (w972:T5)
                        n555 = Unbundle(w972) -> ("2 (CYCLE)"=w969:dbl, "2 (T-RISE min)"=w968:dbl)  [unwired: 4 out]
                        n556 = case shown="\"CYCLE TEST\"" w973 {
                          tunnel: w968 -> [_ _ w980]
                          tunnel: w969 -> [w978 w979 _]
                          tunnel: [w978 w979 w980] -> w971
                          frame "TEST SET UP", Default {
                          }
                          frame "CYCLE TEST" {
                          }
                          frame "T-RISE TEST" {
                          }
                        }
                        n557 = local read "LAB05-2 (TDMS)"() -> (w977:refnum<k34>)
                        n558 = Build Array("STOPPED") -> (w974:string[])
                        n559 = Build Array(w971) -> (w970:dbl[])
                        n560 = TDMS Write(0:w977, 5:"TEST RESULT", 7:w974, 9:w970) -> ()  [unwired: 2 in, 4 out]
                      }
                      frame #1 {
                        n561 = local read "LAB05 (DISP)"() -> (w984:T5)
                        n562 = Bundle(cluster=w984, "2 (STATUS)"="STOP") -> (w983:T5)  [unwired: 5 in]
                        n563 = local write "LAB05-2 (RESULT)"(FALSE) -> ()
                        n564 = local write "LAB05 (DISP)"(w983) -> ()
                      }
                    }
                  }
                  frame True {
                    # "start new test and create test file"
                    n565 = stacked-sequence {
                      seq-local: [w994 _ _ _ _] -> [_ w1013 _ _ _]
                      tunnel: w988 -> [w1003 _ _ _ _]
                      tunnel: w987 -> [w1001 _ _ _ _]
                      tunnel: w986 -> [w1000 _ _ _ _]
                      tunnel: w985 -> [w992 _ _ _ _]
                      frame #0 {
                        n566 = local read "LAB05 (SET)"() -> (w993:T4)
                        n567 = case shown="\"TEST SET UP\", Default" w1000 {
                          tunnel: ["TEST SET UP-" "CYCLE TEST-" "T-RISE TEST-"] -> w996
                          frame "TEST SET UP", Default {
                          }
                          frame "CYCLE TEST" {
                          }
                          frame "T-RISE TEST" {
                          }
                        }
                        n568 = Unbundle(w993) -> ("2 Description"=w989:string)  [unwired: 9 out]
                        n569 = Concatenate Strings(w1003, "LAB05-2\\", w1001, "\\") -> (w997:string)
                        n570 = String To Path(string=w997) -> (path=w999:path)
                        n571 = Concatenate Strings(w997, w996, w989, "-", w992, ".tdms") -> (w994:string)
                        n572 = Create Folder(path (use dialog)=w999) -> (error out=w998:errorcluster)  [unwired: 2 in, 2 out]
                        n573 = call <vilib>:"Clear Errors.vi"("error in (no error)"=w998) -> ()  [unwired: 6 in, 1 out]
                      }
                      frame #1 {
                        n574 = String To Path(string=w1013) -> (path=w1007:path)
                        n575 = TDMS Open(5:FALSE, 6:FALSE, 10:T14."create or replace" ("operation (0:open)"), 11:w1007) -> (0:w1009:errorcluster, 3:→"LAB05-2 (TDMS)":refnum<k34>)  [unwired: 3 in]
                        n576 = local write "data file error"(w1009) -> ()
                      }
                      frame #2 {
                        n577 = local read "LAB05 (SET)"() -> (w1019:T4)
                        n578 = local read "LAB05-2 (TDMS)"() -> (w1030:refnum<k34>)
                        n579 = Build Array("Testers Name", "Description", "Set Test Cycles", "T-Rise minutes", "T-Rise Deg C") -> (w1020:string[])
                        n580 = Unbundle(w1019) -> ("2 Name"=w1018:string, "2 Description"=w1017:string, "2 (CYCLES)"=w1016:dbl, "2 (T-RISE mins)"=w1015:dbl, "2 (T-RISE deg C)"=w1014:dbl)  [unwired: 5 out]
                        n581 = Number To Decimal String(number=w1016) -> (decimal integer string=w1029:string)  [unwired: 1 in]
                        n582 = Number To Decimal String(number=w1015) -> (decimal integer string=w1028:string)  [unwired: 1 in]
                        n583 = Number To Decimal String(number=w1014) -> (decimal integer string=w1027:string)  [unwired: 1 in]
                        n584 = Build Array(w1018, w1017, w1029, w1028, w1027) -> (w1026:string[])
                        n585 = TDMS Set Properties(5:w1026, 7:w1020, 11:w1030) -> ()  [unwired: 3 in, 4 out]
                      }
                      frame #3 {
                        w1032 = 0.0
                        n586 = local read "LAB05 (DISP)"() -> (w1034:T5)
                        n587 = Bundle(cluster=w1034, "2 (CYCLE)"=w1032, "2 (T-RISE min)"=w1032, "2 (STATUS)"="RUN") -> (w1033:T5)  [unwired: 3 in]
                        n588 = local write "LAB05 (DISP)"(w1033) -> ()
                      }
                      frame #4 {
                        n589 = local read "LAB05-2 (SIG)"() -> (w1037:T2)
                        n590 = local read "LAB05 (TEMP START)"() -> (w1039:T6)
                        n591 = Unbundle(w1037) -> ("Tmp Live"=w1036:dbl, "Tmp Neut"=w1035:dbl)  [unwired: 3 out]
                        n592 = Bundle(cluster=w1039, "1 (TL)"=w1036, "1 (TN)"=w1035) -> (w1038:T6)  [unwired: 2 in]
                        n593 = local write "LAB05 (TEMP START)"(w1038) -> ()
                      }
                    }
                  }
                }
              }
            }
          }
          frame #4 {
            # "check if test cycles reached for cycle tests, if so then test pass"
            n594 = stacked-sequence {
              tunnel: w1052 -> [_ _ _ _]
              tunnel: w1051 -> [_ _ _ _]
              tunnel: w1050 -> [_ _ _ _]
              tunnel: w1049 -> [_ _ _ _]
              tunnel: w1048 -> [_ _ _ _]
              tunnel: w1047 -> [_ _ _ _]
              tunnel: w1046 -> [_ _ _ _]
              tunnel: w1045 -> [_ _ _ _]
              tunnel: w1044 -> [_ _ _ _]
              tunnel: w1043 -> [_ _ _ _]
              tunnel: w1042 -> [w1057 _ _ _]
              tunnel: w1041 -> [_ w1089 _ _]
              tunnel: w1040 -> [_ _ w1125 w1162]
              frame #0 {
                # "LAB01-1"
                n595 = Less?(x=w1057, y=2) -> (x < y?=w1055:bool)
                n596 = local read "LAB01 (DISP)"() -> (w1058:T5)
                n597 = Unbundle(w1058) -> ("1 (STATUS)"=w1059:string)  [unwired: 5 out]
                n598 = Equal?(x=w1059, y="RUN") -> (x = y?=w1054:bool)
                n599 = And(x=w1054, y=w1055) -> (x .and. y?=w1053:bool)
                n600 = case shown="True" w1053 {
                  tunnel: w1058 -> [_ w1066]
                  tunnel: w1057 -> [_ w1065]
                  frame False {
                  }
                  frame True {
                    n601 = local read "LAB01 (SET)"() -> (w1068:T4)
                    n602 = Unbundle(w1066) -> ("1 (CYCLE)"=w1067:dbl)  [unwired: 5 out]
                    n603 = Unbundle(w1068) -> ("1 (CYCLES)"=w1062:dbl, "1 (T-RISE mins)"=w1064:dbl)  [unwired: 8 out]
                    n604 = case shown="\"TEST SET UP\", Default" w1065 {
                      tunnel: w1064 -> [_ _ w1075]
                      tunnel: [w1070 w1072 w1075] -> w1063
                      tunnel: w1062 -> [w1070 w1072 _]
                      tunnel: ["TEST SET UP CYCLES" "CYCLES" "T-RISE TEST"] -> w1061
                      frame "TEST SET UP", Default {
                      }
                      frame "CYCLE TEST" {
                      }
                      frame "T-RISE TEST" {
                      }
                    }
                    n605 = Greater Or Equal?(x=w1067, y=w1062) -> (x >= y?=w1069:bool)
                    n606 = case shown="True" w1069 {
                      tunnel: w1063 -> [w1077 _]
                      tunnel: w1061 -> [w1076 _]
                      frame True {
                        n607 = stacked-sequence {
                          tunnel: w1077 -> [w1080 _]
                          tunnel: w1076 -> [w1078 _]
                          frame #0 {
                            n608 = local read "LAB01-1 (TDMS)"() -> (w1084:refnum<k34>)
                            n609 = Build Array(w1078) -> (w1081:string[])
                            n610 = Build Array(w1080) -> (w1079:dbl[])
                            n611 = TDMS Write(0:w1084, 5:"TEST PASS", 7:w1081, 9:w1079) -> (15:w1083:errorcluster)  [unwired: 2 in, 3 out]
                            n612 = local write "data file error"(w1083) -> ()
                          }
                          frame #1 {
                            n613 = local read "LAB01 (DISP)"() -> (w1088:T5)
                            n614 = Bundle(cluster=w1088, "1 (STATUS)"="STOP") -> (w1086:T5)  [unwired: 5 in]
                            n615 = local write "LAB01-1 (RESULT)"(TRUE) -> ()
                            n616 = local write "LAB01 (DISP)"(w1086) -> ()
                          }
                        }
                      }
                      frame False {
                      }
                    }
                  }
                }
              }
              frame #1 {
                # "LAB01-2"
                n617 = Less?(x=w1089, y=2) -> (x < y?=w1093:bool)
                n618 = local read "LAB01 (DISP)"() -> (w1095:T5)
                n619 = Unbundle(w1095) -> ("2 (STATUS)"=w1090:string)  [unwired: 5 out]
                n620 = Equal?(x=w1090, y="RUN") -> (x = y?=w1092:bool)
                n621 = And(x=w1092, y=w1093) -> (x .and. y?=w1091:bool)
                n622 = case shown="True" w1091 {
                  tunnel: w1095 -> [_ w1103]
                  tunnel: w1089 -> [_ w1102]
                  frame False {
                  }
                  frame True {
                    n623 = local read "LAB01 (SET)"() -> (w1104:T4)
                    n624 = Unbundle(w1103) -> ("2 (CYCLE)"=w1099:dbl)  [unwired: 5 out]
                    n625 = Unbundle(w1104) -> ("2 (CYCLES)"=w1097:dbl, "2 (T-RISE mins)"=w1098:dbl)  [unwired: 8 out]
                    n626 = case shown="\"TEST SET UP\", Default" w1102 {
                      tunnel: w1098 -> [_ _ w1111]
                      tunnel: [w1106 w1108 w1111] -> w1101
                      tunnel: w1097 -> [w1106 w1108 _]
                      tunnel: ["TEST SET UP CYCLES" "CYCLES" "T-RISE TEST"] -> w1100
                      frame "TEST SET UP", Default {
                      }
                      frame "CYCLE TEST" {
                      }
                      frame "T-RISE TEST" {
                      }
                    }
                    n627 = Greater Or Equal?(x=w1099, y=w1097) -> (x >= y?=w1105:bool)
                    n628 = case shown="True" w1105 {
                      tunnel: w1101 -> [w1113 _]
                      tunnel: w1100 -> [w1112 _]
                      frame True {
                        n629 = stacked-sequence {
                          tunnel: w1113 -> [w1116 _]
                          tunnel: w1112 -> [w1114 _]
                          frame #0 {
                            n630 = local read "LAB01-2 (TDMS)"() -> (w1120:refnum<k34>)
                            n631 = Build Array(w1114) -> (w1117:string[])
                            n632 = Build Array(w1116) -> (w1115:dbl[])
                            n633 = TDMS Write(0:w1120, 5:"TEST PASS", 7:w1117, 9:w1115) -> (15:w1119:errorcluster)  [unwired: 2 in, 3 out]
                            n634 = local write "data file error"(w1119) -> ()
                          }
                          frame #1 {
                            n635 = local read "LAB01 (DISP)"() -> (w1124:T5)
                            n636 = Bundle(cluster=w1124, "2 (STATUS)"="STOP") -> (w1123:T5)  [unwired: 5 in]
                            n637 = local write "LAB01-2 (RESULT)"(TRUE) -> ()
                            n638 = local write "LAB01 (DISP)"(w1123) -> ()
                          }
                        }
                      }
                      frame False {
                      }
                    }
                  }
                }
              }
              frame #2 {
                # "LAB02-1"
                n639 = Less?(x=w1125, y=2) -> (x < y?=w1129:bool)
                n640 = local read "LAB02 (DISP)"() -> (w1131:T5)
                n641 = Unbundle(w1131) -> ("1 (STATUS)"=w1126:string)  [unwired: 5 out]
                n642 = Equal?(x=w1126, y="RUN") -> (x = y?=w1128:bool)
                n643 = And(x=w1128, y=w1129) -> (x .and. y?=w1127:bool)
                n644 = case shown="True" w1127 {
                  tunnel: w1131 -> [_ w1139]
                  tunnel: w1125 -> [_ w1138]
                  frame False {
                  }
                  frame True {
                    n645 = local read "LAB02 (SET)"() -> (w1140:T4)
                    n646 = Unbundle(w1139) -> ("1 (CYCLE)"=w1135:dbl)  [unwired: 5 out]
                    n647 = Unbundle(w1140) -> ("1 (CYCLES)"=w1134:dbl, "1 (T-RISE mins)"=w1133:dbl)  [unwired: 8 out]
                    n648 = case shown="\"TEST SET UP\", Default" w1138 {
                      tunnel: w1133 -> [_ _ w1147]
                      tunnel: [w1142 w1144 w1147] -> w1137
                      tunnel: w1134 -> [w1142 w1144 _]
                      tunnel: ["TEST SET UP CYCLES" "CYCLES" "T-RISE TEST"] -> w1136
                      frame "TEST SET UP", Default {
                      }
                      frame "CYCLE TEST" {
                      }
                      frame "T-RISE TEST" {
                      }
                    }
                    n649 = Greater Or Equal?(x=w1135, y=w1134) -> (x >= y?=w1141:bool)
                    n650 = case shown="True" w1141 {
                      tunnel: w1137 -> [w1149 _]
                      tunnel: w1136 -> [w1148 _]
                      frame True {
                        n651 = stacked-sequence {
                          tunnel: w1149 -> [w1152 _]
                          tunnel: w1148 -> [w1150 _]
                          frame #0 {
                            n652 = local read "LAB02-1 (TDMS)"() -> (w1156:refnum<k34>)
                            n653 = Build Array(w1150) -> (w1153:string[])
                            n654 = Build Array(w1152) -> (w1151:dbl[])
                            n655 = TDMS Write(0:w1156, 5:"TEST PASS", 7:w1153, 9:w1151) -> (15:w1155:errorcluster)  [unwired: 2 in, 3 out]
                            n656 = local write "data file error"(w1155) -> ()
                          }
                          frame #1 {
                            n657 = local read "LAB02 (DISP)"() -> (w1160:T5)
                            n658 = Bundle(cluster=w1160, "1 (STATUS)"="STOP") -> (w1159:T5)  [unwired: 5 in]
                            n659 = local write "LAB02-1 (RESULT)"(TRUE) -> ()
                            n660 = local write "LAB02 (DISP)"(w1159) -> ()
                          }
                        }
                      }
                      frame False {
                      }
                    }
                  }
                }
              }
              frame #3 {
                # "LAB02-2"
                n661 = Less?(x=w1162, y=2) -> (x < y?=w1165:bool)
                n662 = local read "LAB02 (DISP)"() -> (w1167:T5)
                n663 = Unbundle(w1167) -> ("2 (STATUS)"=w1161:string)  [unwired: 5 out]
                n664 = Equal?(x=w1161, y="RUN") -> (x = y?=w1164:bool)
                n665 = And(x=w1164, y=w1165) -> (x .and. y?=w1163:bool)
                n666 = case shown="True" w1163 {
                  tunnel: w1167 -> [_ w1175]
                  tunnel: w1162 -> [_ w1174]
                  frame False {
                  }
                  frame True {
                    n667 = local read "LAB02 (SET)"() -> (w1176:T4)
                    n668 = Unbundle(w1175) -> ("2 (CYCLE)"=w1171:dbl)  [unwired: 5 out]
                    n669 = Unbundle(w1176) -> ("2 (CYCLES)"=w1169:dbl, "2 (T-RISE mins)"=w1170:dbl)  [unwired: 8 out]
                    n670 = case shown="\"TEST SET UP\", Default" w1174 {
                      tunnel: w1170 -> [_ _ w1183]
                      tunnel: [w1178 w1180 w1183] -> w1173
                      tunnel: w1169 -> [w1178 w1180 _]
                      tunnel: ["TEST SET UP CYCLES" "CYCLES" "T-RISE TEST"] -> w1172
                      frame "TEST SET UP", Default {
                      }
                      frame "CYCLE TEST" {
                      }
                      frame "T-RISE TEST" {
                      }
                    }
                    n671 = Greater Or Equal?(x=w1171, y=w1169) -> (x >= y?=w1177:bool)
                    n672 = case shown="True" w1177 {
                      tunnel: w1173 -> [w1185 _]
                      tunnel: w1172 -> [w1184 _]
                      frame True {
                        n673 = stacked-sequence {
                          tunnel: w1185 -> [w1188 _]
                          tunnel: w1184 -> [w1186 _]
                          frame #0 {
                            n674 = local read "LAB02-2 (TDMS)"() -> (w1192:refnum<k34>)
                            n675 = Build Array(w1186) -> (w1189:string[])
                            n676 = Build Array(w1188) -> (w1187:dbl[])
                            n677 = TDMS Write(0:w1192, 5:"TEST PASS", 7:w1189, 9:w1187) -> (15:w1191:errorcluster)  [unwired: 2 in, 3 out]
                            n678 = local write "data file error"(w1191) -> ()
                          }
                          frame #1 {
                            n679 = local read "LAB02 (DISP)"() -> (w1196:T5)
                            n680 = Bundle(cluster=w1196, "2 (STATUS)"="STOP") -> (w1195:T5)  [unwired: 5 in]
                            n681 = local write "LAB02-2 (RESULT)"(TRUE) -> ()
                            n682 = local write "LAB02 (DISP)"(w1195) -> ()
                          }
                        }
                      }
                      frame False {
                      }
                    }
                  }
                }
              }
            }
          }
          frame #5 {
            # "check if test cycles reached for temperature rise test"
            n683 = stacked-sequence {
              tunnel: w1208 -> [_]
              tunnel: w1207 -> [_]
              tunnel: w1206 -> [_]
              tunnel: w1205 -> [_]
              tunnel: w1204 -> [_]
              tunnel: w1203 -> [_]
              tunnel: w1202 -> [_]
              tunnel: w1201 -> [_]
              tunnel: w1200 -> [_]
              tunnel: w1199 -> [_]
              tunnel: w1198 -> [w1214]
              tunnel: w1197 -> [w1209]
              frame #0 {
                # "LAB01-1"
                n684 = Equal?(x=w1214, y=2) -> (x = y?=w1212:bool)
                n685 = local read "LAB01 (DISP)"() -> (w1215:T5)
                n686 = Unbundle(w1215) -> ("1 (STATUS)"=w1216:string)  [unwired: 5 out]
                n687 = Equal?(x=w1216, y="RUN") -> (x = y?=w1211:bool)
                n688 = And(x=w1211, y=w1212) -> (x .and. y?=w1210:bool)
                n689 = case shown="True" w1210 {
                  tunnel: w1215 -> [_ w1221]
                  tunnel: w1209 -> [_ w1220]
                  frame False {
                  }
                  frame True {
                    n690 = local read "LAB01 (SET)"() -> (w1219:T4)
                    n691 = Unbundle(w1221) -> ("1 (CYCLE)"=w1222:dbl)  [unwired: 5 out]
                    n692 = Unbundle(w1219) -> ("1 (T-RISE mins)"=w1218:dbl)  [unwired: 9 out]
                    n693 = Greater Or Equal?(x=w1222, y=w1220) -> (x >= y?=w1223:bool)
                    n694 = case shown="True" w1223 {
                      tunnel: w1218 -> [w1224 _]
                      frame True {
                        n695 = stacked-sequence {
                          tunnel: w1224 -> [w1226 _]
                          frame #0 {
                            n696 = local read "LAB01-1 (TDMS)"() -> (w1231:refnum<k34>)
                            n697 = Build Array("T-RISE") -> (w1228:string[])
                            n698 = Build Array(w1226) -> (w1227:dbl[])
                            n699 = TDMS Write(0:w1231, 5:"TEST PASS", 7:w1228, 9:w1227) -> (15:w1230:errorcluster)  [unwired: 2 in, 3 out]
                            n700 = local write "data file error"(w1230) -> ()
                          }
                          frame #1 {
                            n701 = local read "LAB01 (DISP)"() -> (w1235:T5)
                            n702 = Bundle(cluster=w1235, "1 (STATUS)"="STOP") -> (w1233:T5)  [unwired: 5 in]
                            n703 = local write "LAB01-1 (RESULT)"(TRUE) -> ()
                            n704 = local write "LAB01 (DISP)"(w1233) -> ()
                          }
                        }
                      }
                      frame False {
                      }
                    }
                  }
                }
              }
            }
          }
          frame #6 {
            # "disable functions"
            n705 = stacked-sequence {
              tunnel: w1245 -> [w1255 _ w1305]
              tunnel: w1244 -> [w1254 _ w1304]
              tunnel: w1243 -> [w1253 _ w1303]
              tunnel: w1242 -> [w1252 _ w1302]
              tunnel: w1241 -> [w1251 _ w1301]
              tunnel: w1240 -> [_ w1275 w1300]
              tunnel: w1239 -> [_ w1274 w1299]
              tunnel: w1238 -> [_ w1273 w1298]
              tunnel: w1237 -> [_ w1272 w1297]
              tunnel: w1236 -> [_ w1271 w1296]
              frame #0 {
                n706 = Select(t=2, s=w1252, f=0) -> (s? t:f=w1247:i32)
                n707 = Select(t=2, s=w1253, f=0) -> (s? t:f=w1248:i32)
                n708 = Select(t=2, s=w1251, f=0) -> (s? t:f=w1246:i32)
                n709 = Select(t=2, s=w1255, f=0) -> (s? t:f=w1250:i32)
                n710 = Select(t=2, s=w1254, f=0) -> (s? t:f=w1249:i32)
                n711 = property on="LAB02-2 SELECT" class="RadioBtnsControl (strict)"("DisabledEnum"=w1247) -> ()  [unwired: 2 in, 2 out]
                n712 = property on="LAB02-1 SELECT" class="RadioBtnsControl (strict)"("DisabledEnum"=w1248) -> ()  [unwired: 2 in, 2 out]
                n713 = property on="LAB03-1 SELECT" class="RadioBtnsControl (strict)"("DisabledEnum"=w1246) -> ()  [unwired: 2 in, 2 out]
                n714 = property on="LAB01-1 SELECT" class="RadioBtnsControl (strict)"("DisabledEnum"=w1250) -> ()  [unwired: 2 in, 2 out]
                n715 = property on="LAB01-2 SELECT" class="RadioBtnsControl (strict)"("DisabledEnum"=w1249) -> ()  [unwired: 2 in, 2 out]
                n716 = property on="LAB01-2 (RESULT)" class="Bool (strict)"("DisabledEnum"=w1249) -> ()  [unwired: 2 in, 2 out]
                n717 = property on="LAB02-1 (RESULT)" class="Bool (strict)"("DisabledEnum"=w1248) -> ()  [unwired: 2 in, 2 out]
                n718 = property on="LAB01-1 (RESULT)" class="Bool (strict)"("DisabledEnum"=w1250) -> ()  [unwired: 2 in, 2 out]
                n719 = property on="LAB02-2 (RESULT)" class="Bool (strict)"("DisabledEnum"=w1247) -> ()  [unwired: 2 in, 2 out]
                n720 = property on="LAB03-1 (RESULT)" class="Bool (strict)"("DisabledEnum"=w1246) -> ()  [unwired: 2 in, 2 out]
              }
              frame #1 {
                n721 = Select(t=2, s=w1271, f=0) -> (s? t:f=w1266:i32)
                n722 = Select(t=2, s=w1272, f=0) -> (s? t:f=w1267:i32)
                n723 = Select(t=2, s=w1275, f=0) -> (s? t:f=w1270:i32)
                n724 = Select(t=2, s=w1274, f=0) -> (s? t:f=w1269:i32)
                n725 = Select(t=2, s=w1273, f=0) -> (s? t:f=w1268:i32)
                n726 = property on="LAB05-2 SELECT" class="RadioBtnsControl (strict)"("DisabledEnum"=w1266) -> ()  [unwired: 2 in, 2 out]
                n727 = property on="LAB05-1 SELECT" class="RadioBtnsControl (strict)"("DisabledEnum"=w1267) -> ()  [unwired: 2 in, 2 out]
                n728 = property on="LAB03-2 SELECT" class="RadioBtnsControl (strict)"("DisabledEnum"=w1270) -> ()  [unwired: 2 in, 2 out]
                n729 = property on="LAB04-1 SELECT" class="RadioBtnsControl (strict)"("DisabledEnum"=w1269) -> ()  [unwired: 2 in, 2 out]
                n730 = property on="LAB04-2 SELECT" class="RadioBtnsControl (strict)"("DisabledEnum"=w1268) -> ()  [unwired: 2 in, 2 out]
                n731 = property on="LAB05-2 (RESULT)" class="Bool (strict)"("DisabledEnum"=w1266) -> ()  [unwired: 2 in, 2 out]
                n732 = property on="LAB05-1 (RESULT)" class="Bool (strict)"("DisabledEnum"=w1267) -> ()  [unwired: 2 in, 2 out]
                n733 = property on="LAB04-2 (RESULT)" class="Bool (strict)"("DisabledEnum"=w1268) -> ()  [unwired: 2 in, 2 out]
                n734 = property on="LAB04-1 (RESULT)" class="Bool (strict)"("DisabledEnum"=w1269) -> ()  [unwired: 2 in, 2 out]
                n735 = property on="LAB03-2 (RESULT)" class="Bool (strict)"("DisabledEnum"=w1270) -> ()  [unwired: 2 in, 2 out]
              }
              frame #2 {
                # "disable calibrate if any test running"
                n736 = Or(x=w1297, y=w1296) -> (x .or. y?=w1290:bool)
                n737 = Or(x=w1299, y=w1298) -> (x .or. y?=w1292:bool)
                n738 = Or(x=w1303, y=w1302) -> (x .or. y?=w1294:bool)
                n739 = Or(x=w1301, y=w1300) -> (x .or. y?=w1293:bool)
                n740 = Or(x=w1305, y=w1304) -> (x .or. y?=w1295:bool)
                n741 = Or(x=w1293, y=w1292) -> (x .or. y?=w1291:bool)
                n742 = Or(x=w1295, y=w1294) -> (x .or. y?=w1289:bool)
                n743 = Or(x=w1291, y=w1290) -> (x .or. y?=w1288:bool)
                n744 = Or(x=w1289, y=w1288) -> (x .or. y?=w1287:bool)
                n745 = case shown="False" w1287 {
                  tunnel: [0 2] -> w1286
                  frame False {
                  }
                  frame True {
                  }
                }
                n746 = property on="CALIBRATE" class="Bool (strict)"("DisabledEnum"=w1286) -> ()  [unwired: 2 in, 2 out]
              }
            }
          }
          frame #7 {
            # "end test & close test files"
            n747 = stacked-sequence {
              frame #0 {
                n748 = local read "LAB01 (DISP)"() -> (w1309:T5)
                n749 = Unbundle(w1309) -> ("1 (STATUS)"=w1308:string)  [unwired: 5 out]
                n750 = Equal?(x=w1308, y="STOP") -> (x = y?=w1310:bool)
                n751 = case shown="True" w1310 {
                  frame False {
                  }
                  frame True {
                    n752 = stacked-sequence {
                      frame #0 {
                        n753 = local read "LAB01 (DISP)"() -> (w1314:T5)
                        n754 = Bundle(cluster=w1314, "1 (STATUS)"="END") -> (w1312:T5)  [unwired: 5 in]
                        n755 = local write "LAB01 (DISP)"(w1312) -> ()
                      }
                      frame #1 {
                        n756 = local read "LAB01-1 (TDMS)"() -> (w1317:refnum<k34>)
                        n757 = TDMS Close(11:w1317) -> (0:w1316:errorcluster)  [unwired: 1 in, 1 out]
                        n758 = local write "LAB01-1RUN"(FALSE) -> ()
                        n759 = local write "data file error"(w1316) -> ()
                      }
                    }
                  }
                }
              }
            }
          }
          frame #8 {
            # "drive jigs"
            n760 = stacked-sequence {
              frame #0 {
                # "jig on"
                n761 = local read "jig cycle"() -> (w1318:dbl)
                n762 = Equal?(x=w1318, y=0) -> (x = y?=w1320:bool)
                n763 = case shown="True" w1320 {
                  frame False {
                  }
                  frame True {
                    n764 = local read "LAB01-1RUN"() -> (w1321:bool)
                    n765 = local read "LAB01-2 RUN"() -> (w1322:bool)
                    n766 = local read "LAB03-1 RUN"() -> (w1328:bool)
                    n767 = local read "LAB03-2 RUN"() -> (w1327:bool)
                    n768 = local read "LAB02-1 RUN"() -> (w1330:bool)
                    n769 = local read "LAB02-2 RUN"() -> (w1329:bool)
                    n770 = local read "LAB04-1 RUN"() -> (w1326:bool)
                    n771 = local read "LAB04-2 RUN"() -> (w1325:bool)
                    n772 = local read "LAB05-1 RUN"() -> (w1324:bool)
                    n773 = local read "LAB05-2 RUN"() -> (w1323:bool)
                    n774 = local write "LAB05-1 (JIG)"(w1324) -> ()
                    n775 = local write "LAB05-2 (JIG)"(w1323) -> ()
                    n776 = local write "LAB04-2 (JIG)"(w1325) -> ()
                    n777 = local write "LAB02-1 (JIG)"(w1330) -> ()
                    n778 = local write "LAB03-1 (JIG)"(w1328) -> ()
                    n779 = local write "LAB04-1 (JIG)"(w1326) -> ()
                    n780 = local write "LAB03-2 (JIG)"(w1327) -> ()
                    n781 = local write "LAB02-2 (JIG)"(w1329) -> ()
                    n782 = local write "LAB01-1 (JIG)"(w1321) -> ()
                    n783 = local write "LAB01-2 (JIG)"(w1322) -> ()
                  }
                }
              }
              frame #1 {
                # "jig off"
                n784 = local read "jig cycle"() -> (w1333:dbl)
                n785 = local read "on loops"() -> (w1332:dbl)
                n786 = Equal?(x=w1333, y=w1332) -> (x = y?=w1331:bool)
                n787 = case shown="True" w1331 {
                  frame False {
                  }
                  frame True {
                    w1384 = FALSE
                    w1385 = TRUE
                    w1383 = 2
                    n788 = local read "LAB05-2 SELECT"() -> (w1374:T3)
                    n789 = local read "LAB04-2 SELECT"() -> (w1376:T3)
                    n790 = local read "LAB04-1 SELECT"() -> (w1377:T3)
                    n791 = local read "LAB05-1 SELECT"() -> (w1375:T3)
                    n792 = local read "LAB03-2 SELECT"() -> (w1378:T3)
                    n793 = local read "LAB02-1 SELECT"() -> (w1381:T3)
                    n794 = local read "LAB03-1 SELECT"() -> (w1379:T3)
                    n795 = local read "LAB02-2 SELECT"() -> (w1380:T3)
                    n796 = local read "LAB01-2 SELECT"() -> (w1382:T3)
                    n797 = local read "LAB05-1 RUN"() -> (w1344:bool)
                    n798 = local read "LAB05-2 RUN"() -> (w1343:bool)
                    n799 = local read "LAB04-2 RUN"() -> (w1345:bool)
                    n800 = local read "LAB04-1 RUN"() -> (w1346:bool)
                    n801 = local read "LAB01-2 RUN"() -> (w1351:bool)
                    n802 = local read "LAB03-2 RUN"() -> (w1347:bool)
                    n803 = local read "LAB01-1RUN"() -> (w1362:bool)
                    n804 = local read "LAB01-1 SELECT"() -> (w1386:T3)
                    n805 = local read "LAB03-1 RUN"() -> (w1348:bool)
                    n806 = local read "LAB02-1 RUN"() -> (w1350:bool)
                    n807 = local read "LAB02-2 RUN"() -> (w1349:bool)
                    n808 = Equal?(x=w1383, y=w1379) -> (x = y?=w1357:bool)
                    n809 = Equal?(x=w1383, y=w1378) -> (x = y?=w1356:bool)
                    n810 = Equal?(x=w1383, y=w1377) -> (x = y?=w1355:bool)
                    n811 = Equal?(x=w1383, y=w1376) -> (x = y?=w1354:bool)
                    n812 = Equal?(x=w1383, y=w1375) -> (x = y?=w1353:bool)
                    n813 = Equal?(x=w1383, y=w1374) -> (x = y?=w1352:bool)
                    n814 = Equal?(x=w1383, y=w1386) -> (x = y?=w1363:bool)
                    n815 = Equal?(x=w1383, y=w1381) -> (x = y?=w1359:bool)
                    n816 = Equal?(x=w1383, y=w1380) -> (x = y?=w1358:bool)
                    n817 = Equal?(x=w1383, y=w1382) -> (x = y?=w1360:bool)
                    n818 = And(x=w1354, y=w1345) -> (x .and. y?=w1336:bool)
                    n819 = And(x=w1357, y=w1348) -> (x .and. y?=w1339:bool)
                    n820 = And(x=w1355, y=w1346) -> (x .and. y?=w1337:bool)
                    n821 = And(x=w1352, y=w1343) -> (x .and. y?=w1334:bool)
                    n822 = And(x=w1358, y=w1349) -> (x .and. y?=w1340:bool)
                    n823 = And(x=w1356, y=w1347) -> (x .and. y?=w1338:bool)
                    n824 = And(x=w1353, y=w1344) -> (x .and. y?=w1335:bool)
                    n825 = And(x=w1360, y=w1351) -> (x .and. y?=w1342:bool)
                    n826 = And(x=w1363, y=w1362) -> (x .and. y?=w1361:bool)
                    n827 = And(x=w1359, y=w1350) -> (x .and. y?=w1341:bool)
                    n828 = Select(t=w1385, s=w1361, f=w1384) -> (s? t:f=w1364:bool)
                    n829 = Select(t=w1385, s=w1342, f=w1384) -> (s? t:f=w1365:bool)
                    n830 = Select(t=w1385, s=w1341, f=w1384) -> (s? t:f=w1366:bool)
                    n831 = Select(t=w1385, s=w1340, f=w1384) -> (s? t:f=w1367:bool)
                    n832 = Select(t=w1385, s=w1339, f=w1384) -> (s? t:f=w1368:bool)
                    n833 = Select(t=w1385, s=w1338, f=w1384) -> (s? t:f=w1369:bool)
                    n834 = Select(t=w1385, s=w1337, f=w1384) -> (s? t:f=w1370:bool)
                    n835 = Select(t=w1385, s=w1336, f=w1384) -> (s? t:f=w1371:bool)
                    n836 = Select(t=w1385, s=w1335, f=w1384) -> (s? t:f=w1372:bool)
                    n837 = Select(t=w1385, s=w1334, f=w1384) -> (s? t:f=w1373:bool)
                    n838 = local write "LAB03-2 (JIG)"(w1369) -> ()
                    n839 = local write "LAB02-1 (JIG)"(w1366) -> ()
                    n840 = local write "LAB02-2 (JIG)"(w1367) -> ()
                    n841 = local write "LAB01-2 (JIG)"(w1365) -> ()
                    n842 = local write "LAB03-1 (JIG)"(w1368) -> ()
                    n843 = local write "LAB01-1 (JIG)"(w1364) -> ()
                    n844 = local write "LAB05-2 (JIG)"(w1373) -> ()
                    n845 = local write "LAB04-1 (JIG)"(w1370) -> ()
                    n846 = local write "LAB05-1 (JIG)"(w1372) -> ()
                    n847 = local write "LAB04-2 (JIG)"(w1371) -> ()
                  }
                }
              }
            }
          }
          frame #9 {
            # "drive digital output"
            n848 = local read "LAB05-2 (O/I)"() -> (w1392:bool)
            n849 = local read "LAB05-2 (JIG)"() -> (w1391:bool)
            n850 = local read "LAB05-1 (O/I)"() -> (w1394:bool)
            n851 = local read "LAB05-1 (JIG)"() -> (w1393:bool)
            n852 = local read "LAB04-2 (O/I)"() -> (w1396:bool)
            n853 = local read "LAB04-2 (JIG)"() -> (w1395:bool)
            n854 = local read "LAB03-1 (O/I)"() -> (w1401:bool)
            n855 = local read "LAB04-1 (O/I)"() -> (w1397:bool)
            n856 = local read "LAB04-1 (JIG)"() -> (w1390:bool)
            n857 = local read "LAB02-1 (O/I)"() -> (w1405:bool)
            n858 = local read "LAB02-2 (O/I)"() -> (w1403:bool)
            n859 = local read "LAB03-2 (O/I)"() -> (w1399:bool)
            n860 = local read "LAB03-2 (JIG)"() -> (w1398:bool)
            n861 = local read "LAB02-1 (JIG)"() -> (w1404:bool)
            n862 = local read "LAB02-2 (JIG)"() -> (w1402:bool)
            n863 = local read "LAB03-1 (JIG)"() -> (w1400:bool)
            n864 = local read "LAB01-2 (O/I)"() -> (w1407:bool)
            n865 = local read "LAB01-2 (JIG)"() -> (w1406:bool)
            n866 = local read "LAB01-1 (O/I)"() -> (w1409:bool)
            n867 = local read "LAB01-1 (JIG)"() -> (w1408:bool)
            n868 = Build Array(w1396, w1395, w1394, w1393, w1392, w1391) -> (w1387:bool[])
            n869 = Build Array(w1402, w1401, w1400, w1399, w1398, w1397, w1390) -> (w1388:bool[])
            n870 = Build Array(w1409, w1408, w1407, w1406, w1405, w1404, w1403) -> (w1389:bool[])
            n871 = call "sub vi - Drive Relays All v6.vi"("Array #2"=w1387, "Array #1"=w1388, "Array #0"=w1389) -> ()  [unwired: 8 in, 1 out]
          }
          frame #10 {
            # "get temperature values"
            n872 = stacked-sequence {
              frame #0 {
                n873 = local read "jig cycle"() -> (w1410:dbl)
                n874 = local read "on loops"() -> (w1413:dbl)
                n875 = local read "jig cycle"() -> (w1415:dbl)
                n876 = Add(x=w1413, y=1) -> (x+y=w1414:dbl)
                n877 = Equal?(x=w1415, y=0) -> (x = y?=w1416:bool)
                n878 = Equal?(x=w1410, y=w1414) -> (x = y?=w1411:bool)
                n879 = case shown="True" w1416 {
                  frame False {
                  }
                  frame True {
                    w1428 = FALSE
                    w1429 = TRUE
                    n880 = local write "TEMP update"(TRUE) -> ()
                    n881 = call "sub vi - GET ALL TEMP v3.vi"("LA01-EN"=w1429, "LA02-EN"=w1429, "LA03-EN"=w1429, "LA04-EN"=w1428, "LA05-EN"=w1428, "Gen Cal Value"=1.0) -> ("LA01 TEMP"=w1427:T15, "LA02 TEMP"=w1425:T15, "LA03 TEMP"=w1424:T15)  [unwired: 4 in, 3 out]
                    n882 = local write "LAB03 TEMP"(w1424) -> ()
                    n883 = local write "LAB02 TEMP"(w1425) -> ()
                    n884 = local write "LAB01 TEMP"(w1427) -> ()
                  }
                }
                n885 = case shown="True" w1411 {
                  frame False {
                  }
                  frame True {
                    w1421 = TRUE
                    w1422 = FALSE
                    n886 = local write "TEMP update"(TRUE) -> ()
                    n887 = call "sub vi - GET ALL TEMP v3.vi"("LA01-EN"=w1422, "LA02-EN"=w1422, "LA03-EN"=w1422, "LA04-EN"=w1421, "LA05-EN"=w1421, "Gen Cal Value"=1.0) -> ("LA04 TEMP"=w1419:T15, "LA05 TEMP"=w1418:T15)  [unwired: 4 in, 4 out]
                    n888 = local write "LAB04 TEMP"(w1419) -> ()
                    n889 = local write "LAB05 TEMP"(w1418) -> ()
                  }
                }
              }
              frame #1 {
                n890 = local read "LAB01 (CAL)"() -> (w1447:T7)
                n891 = local read "LAB01 TEMP"() -> (w1448:T10)
                n892 = Unbundle By Name(w1448) -> ("T1 Live"=w1438:dbl, "T1 Neut"=w1437:dbl, "T2 Live"=w1436:dbl, "T2 Neut"=w1435:dbl)  [unwired: 2 out]
                n893 = Unbundle By Name(w1447) -> ("1 (TL) cal"=w1434:dbl, "1 (TN) cal"=w1433:dbl, "2 (TL) cal"=w1432:dbl, "2 (TN) cal"=w1431:dbl)  [unwired: 6 out]
                n894 = Multiply(x=w1438, y=w1434) -> (x*y=w1444:dbl)
                n895 = Multiply(x=w1437, y=w1433) -> (x*y=w1443:dbl)
                n896 = Multiply(x=w1436, y=w1432) -> (x*y=w1440:dbl)
                n897 = Multiply(x=w1435, y=w1431) -> (x*y=w1439:dbl)
                n898 = local read "LAB01-2 (SIG)"() -> (w1442:T2)
                n899 = local read "LAB01-1 (SIG)"() -> (w1446:T2)
                n900 = Bundle By Name(cluster=w1446, "Tmp Live"=w1444, "Tmp Neut"=w1443) -> (w1445:T2)
                n901 = Bundle By Name(cluster=w1442, "Tmp Live"=w1440, "Tmp Neut"=w1439) -> (w1441:T2)
                n902 = local write "LAB01-1 (SIG)"(w1445) -> ()
                n903 = local write "LAB01-2 (SIG)"(w1441) -> ()
              }
              frame #2 {
                n904 = local read "LAB02 (CAL)"() -> (w1465:T8)
                n905 = local read "LAB02 TEMP"() -> (w1466:T10)
                n906 = Unbundle By Name(w1466) -> ("T1 Live"=w1456:dbl, "T1 Neut"=w1455:dbl, "T2 Live"=w1454:dbl, "T2 Neut"=w1453:dbl)  [unwired: 2 out]
                n907 = Unbundle By Name(w1465) -> ("1 (TL) cal"=w1452:dbl, "1 (TN) cal"=w1451:dbl, "2 (TL) cal"=w1450:dbl, "2 (TN) cal"=w1449:dbl)  [unwired: 6 out]
                n908 = Multiply(x=w1456, y=w1452) -> (x*y=w1462:dbl)
                n909 = Multiply(x=w1455, y=w1451) -> (x*y=w1461:dbl)
                n910 = Multiply(x=w1454, y=w1450) -> (x*y=w1458:dbl)
                n911 = Multiply(x=w1453, y=w1449) -> (x*y=w1457:dbl)
                n912 = local read "LAB02-2 (SIG)"() -> (w1460:T2)
                n913 = local read "LAB02-1 (SIG)"() -> (w1464:T2)
                n914 = Bundle By Name(cluster=w1464, "Tmp Live"=w1462, "Tmp Neut"=w1461) -> (w1463:T2)
                n915 = Bundle By Name(cluster=w1460, "Tmp Live"=w1458, "Tmp Neut"=w1457) -> (w1459:T2)
                n916 = local write "LAB02-1 (SIG)"(w1463) -> ()
                n917 = local write "LAB02-2 (SIG)"(w1459) -> ()
              }
              frame #3 {
                n918 = local read "LAB03 (CAL)"() -> (w1483:T7)
                n919 = local read "LAB03 TEMP"() -> (w1484:T10)
                n920 = Unbundle By Name(w1484) -> ("T1 Live"=w1474:dbl, "T1 Neut"=w1473:dbl, "T2 Live"=w1472:dbl, "T2 Neut"=w1471:dbl)  [unwired: 2 out]
                n921 = Unbundle By Name(w1483) -> ("1 (TL) cal"=w1470:dbl, "1 (TN) cal"=w1469:dbl, "2 (TL) cal"=w1468:dbl, "2 (TN) cal"=w1467:dbl)  [unwired: 6 out]
                n922 = Multiply(x=w1474, y=w1470) -> (x*y=w1480:dbl)
                n923 = Multiply(x=w1473, y=w1469) -> (x*y=w1479:dbl)
                n924 = Multiply(x=w1472, y=w1468) -> (x*y=w1476:dbl)
                n925 = Multiply(x=w1471, y=w1467) -> (x*y=w1475:dbl)
                n926 = local read "LAB03-2 (SIG)"() -> (w1478:T2)
                n927 = local read "LAB03-1 (SIG)"() -> (w1482:T2)
                n928 = Bundle By Name(cluster=w1482, "Tmp Live"=w1480, "Tmp Neut"=w1479) -> (w1481:T2)
                n929 = Bundle By Name(cluster=w1478, "Tmp Live"=w1476, "Tmp Neut"=w1475) -> (w1477:T2)
                n930 = local write "LAB03-1 (SIG)"(w1481) -> ()
                n931 = local write "LAB03-2 (SIG)"(w1477) -> ()
              }
              frame #4 {
                n932 = local read "LAB04 (CAL)"() -> (w1501:T7)
                n933 = local read "LAB04 TEMP"() -> (w1502:T10)
                n934 = Unbundle By Name(w1502) -> ("T1 Live"=w1492:dbl, "T1 Neut"=w1491:dbl, "T2 Live"=w1490:dbl, "T2 Neut"=w1489:dbl)  [unwired: 2 out]
                n935 = Unbundle By Name(w1501) -> ("1 (TL) cal"=w1488:dbl, "1 (TN) cal"=w1487:dbl, "2 (TL) cal"=w1486:dbl, "2 (TN) cal"=w1485:dbl)  [unwired: 6 out]
                n936 = Multiply(x=w1492, y=w1488) -> (x*y=w1498:dbl)
                n937 = Multiply(x=w1491, y=w1487) -> (x*y=w1497:dbl)
                n938 = Multiply(x=w1490, y=w1486) -> (x*y=w1494:dbl)
                n939 = Multiply(x=w1489, y=w1485) -> (x*y=w1493:dbl)
                n940 = local read "LAB04-2 (SIG)"() -> (w1496:T2)
                n941 = local read "LAB04-1 (SIG)"() -> (w1500:T2)
                n942 = Bundle By Name(cluster=w1500, "Tmp Live"=w1498, "Tmp Neut"=w1497) -> (w1499:T2)
                n943 = Bundle By Name(cluster=w1496, "Tmp Live"=w1494, "Tmp Neut"=w1493) -> (w1495:T2)
                n944 = local write "LAB04-1 (SIG)"(w1499) -> ()
                n945 = local write "LAB04-2 (SIG)"(w1495) -> ()
              }
              frame #5 {
                n946 = local read "LAB05 (CAL)"() -> (w1519:T7)
                n947 = local read "LAB05 TEMP"() -> (w1520:T10)
                n948 = Unbundle By Name(w1520) -> ("T1 Live"=w1510:dbl, "T1 Neut"=w1509:dbl, "T2 Live"=w1508:dbl, "T2 Neut"=w1507:dbl)  [unwired: 2 out]
                n949 = Unbundle By Name(w1519) -> ("1 (TL) cal"=w1506:dbl, "1 (TN) cal"=w1505:dbl, "2 (TL) cal"=w1504:dbl, "2 (TN) cal"=w1503:dbl)  [unwired: 6 out]
                n950 = Multiply(x=w1510, y=w1506) -> (x*y=w1516:dbl)
                n951 = Multiply(x=w1509, y=w1505) -> (x*y=w1515:dbl)
                n952 = Multiply(x=w1508, y=w1504) -> (x*y=w1512:dbl)
                n953 = Multiply(x=w1507, y=w1503) -> (x*y=w1511:dbl)
                n954 = local read "LAB05-2 (SIG)"() -> (w1514:T2)
                n955 = local read "LAB05-1 (SIG)"() -> (w1518:T2)
                n956 = Bundle By Name(cluster=w1518, "Tmp Live"=w1516, "Tmp Neut"=w1515) -> (w1517:T2)
                n957 = Bundle By Name(cluster=w1514, "Tmp Live"=w1512, "Tmp Neut"=w1511) -> (w1513:T2)
                n958 = local write "LAB05-1 (SIG)"(w1517) -> ()
                n959 = local write "LAB05-2 (SIG)"(w1513) -> ()
              }
            }
          }
          frame #11 {
            # "get analog values"
            n960 = local read "on loops"() -> (w1527:dbl)
            n961 = local read "jig cycle"() -> (w1524:dbl)
            n962 = Add(x=w1527, y=2) -> (x+y=w1525:dbl)
            n963 = Equal?(x=w1524, y=1) -> (x = y?=w1522:bool)
            n964 = Equal?(x=w1524, y=w1525) -> (x = y?=w1523:bool)
            n965 = Or(x=w1522, y=w1523) -> (x .or. y?=w1521:bool)
            n966 = case shown="True" w1521 {
              frame False {
              }
              frame True {
                n967 = call "sub vi - Read Analog All v7.vi"() -> ("Analog loop time"=w1535:dbl, "array GRAPH"=w1534:dynamicdata[], "LAB01"=w1533:T16, "LAB02"=w1532:T17, "LAB03"=w1531:T18, "LAB04"=w1530:T19, "array ERROR"=w1536:errorcluster[], "LAB05"=w1529:T20)  [unwired: 8 in]
                n968 = stacked-sequence {
                  tunnel: w1536 -> [w1539 _ _ _ _ _]
                  tunnel: w1535 -> [w1538 _ _ _ _ _]
                  tunnel: w1534 -> [w1537 _ _ _ _ _]
                  tunnel: w1533 -> [_ w1584 _ _ _ _]
                  tunnel: w1532 -> [_ _ w1585 _ _ _]
                  tunnel: w1531 -> [_ _ _ w1609 _ _]
                  tunnel: w1530 -> [_ _ _ _ w1633 _]
                  tunnel: w1529 -> [_ _ _ _ _ w1657]
                  frame #0 {
                    n969 = local write "AI update"(TRUE) -> ()
                    n970 = Index Array(array=w1537, index=6) -> (element=→"LAB04-1 (GRAPH)":dynamicdata)
                    n971 = Index Array(array=w1537, index=7) -> (element=→"LAB04-2 (GRAPH)":dynamicdata)
                    n972 = Index Array(array=w1537, index=9) -> (element=→"LAB05-2 (GRAPH)":dynamicdata)
                    n973 = Index Array(array=w1537, index=8) -> (element=→"LAB05-1 (GRAPH)":dynamicdata)
                    n974 = Index Array(array=w1537, index=5) -> (element=→"LAB03-2 (GRAPH)":dynamicdata)
                    n975 = Index Array(array=w1537, index=0) -> (element=→"LAB01-1 (GRAPH)":dynamicdata)
                    n976 = Index Array(array=w1537, index=1) -> (element=→"LAB01-2 (GRAPH)":dynamicdata)
                    n977 = Index Array(array=w1537, index=2) -> (element=→"LAB02-1 (GRAPH)":dynamicdata)
                    n978 = Index Array(array=w1537, index=3) -> (element=→"LAB02-2 (GRAPH)":dynamicdata)
                    n979 = Index Array(array=w1537, index=4) -> (element=→"LAB03-1 (GRAPH)":dynamicdata)
                    "AI loop time" <- w1538
                    "Analog Error Array" <- w1539
                  }
                  frame #1 {
                    n980 = local read "LAB01 (CAL)"() -> (w1583:T7)
                    n981 = Unbundle By Name(w1584) -> ("LAB01-1 (A)"=w1582:dbl, "LAB01-1 (V)"=w1581:dbl, "LAB01-1 (PF)"=w1580:dbl, "LAB01-2 (A)"=w1579:dbl, "LAB01-2 (V)"=w1578:dbl, "LAB01-2 (PF)"=w1577:dbl)
                    n982 = Unbundle By Name(w1583) -> ("1  (A) cal"=w1576:dbl, "1 (V) cal"=w1575:dbl, "1 (PF) cal"=w1574:dbl, "2 (A) cal"=w1573:dbl, "2 (V) cal"=w1572:dbl, "2 (PF) cal"=w1571:dbl)  [unwired: 4 out]
                    n983 = Multiply(x=w1582, y=w1576) -> (x*y=w1569:dbl)
                    n984 = Multiply(x=w1581, y=w1575) -> (x*y=w1568:dbl)
                    n985 = Multiply(x=w1580, y=w1574) -> (x*y=w1567:dbl)
                    n986 = Multiply(x=w1579, y=w1573) -> (x*y=w1563:dbl)
                    n987 = local read "LAB01-1 (SIG)"() -> (w1570:T2)
                    n988 = Multiply(x=w1578, y=w1572) -> (x*y=w1562:dbl)
                    n989 = Multiply(x=w1577, y=w1571) -> (x*y=w1561:dbl)
                    n990 = local read "LAB01-2 (SIG)"() -> (w1565:T2)
                    n991 = Bundle By Name(cluster=w1570, "AMPS"=w1569, "VOLTS"=w1568, "PF"=w1567) -> (w1566:T2)
                    n992 = Bundle By Name(cluster=w1565, "AMPS"=w1563, "VOLTS"=w1562, "PF"=w1561) -> (w1564:T2)
                    n993 = local write "LAB01-2 (SIG)"(w1564) -> ()
                    n994 = local write "LAB01-1 (SIG)"(w1566) -> ()
                  }
                  frame #2 {
                    n995 = local read "LAB02 (CAL)"() -> (w1608:T8)
                    n996 = Unbundle By Name(w1585) -> ("LAB02-1 (A)"=w1607:dbl, "LAB02-1 (V)"=w1606:dbl, "LAB02-1 (PF)"=w1605:dbl, "LAB02-2 (A)"=w1604:dbl, "LAB02-2 (V)"=w1603:dbl, "LAB02-2 (PF)"=w1602:dbl)
                    n997 = Unbundle By Name(w1608) -> ("1 (A) cal"=w1601:dbl, "1 (V) cal"=w1600:dbl, "1 (PF) cal"=w1599:dbl, "2 (A) cal"=w1598:dbl, "2 (V) cal"=w1597:dbl, "2 (PF) cal"=w1596:dbl)  [unwired: 4 out]
                    n998 = Multiply(x=w1607, y=w1601) -> (x*y=w1594:dbl)
                    n999 = Multiply(x=w1606, y=w1600) -> (x*y=w1593:dbl)
                    n1000 = Multiply(x=w1605, y=w1599) -> (x*y=w1592:dbl)
                    n1001 = Multiply(x=w1604, y=w1598) -> (x*y=w1588:dbl)
                    n1002 = local read "LAB02-1 (SIG)"() -> (w1595:T2)
                    n1003 = Multiply(x=w1603, y=w1597) -> (x*y=w1587:dbl)
                    n1004 = Multiply(x=w1602, y=w1596) -> (x*y=w1586:dbl)
                    n1005 = local read "LAB02-2 (SIG)"() -> (w1590:T2)
                    n1006 = Bundle By Name(cluster=w1595, "AMPS"=w1594, "VOLTS"=w1593, "PF"=w1592) -> (w1591:T2)
                    n1007 = Bundle By Name(cluster=w1590, "AMPS"=w1588, "VOLTS"=w1587, "PF"=w1586) -> (w1589:T2)
                    n1008 = local write "LAB02-2 (SIG)"(w1589) -> ()
                    n1009 = local write "LAB02-1 (SIG)"(w1591) -> ()
                  }
                  frame #3 {
                    n1010 = local read "LAB03 (CAL)"() -> (w1632:T7)
                    n1011 = Unbundle By Name(w1609) -> ("LAB03-1 (A)"=w1631:dbl, "LAB03-1 (V)"=w1630:dbl, "LAB03-1 (PF)"=w1629:dbl, "LAB03-2 (A)"=w1628:dbl, "LAB03-2 (V)"=w1627:dbl, "LAB03-2 (PF)"=w1626:dbl)
                    n1012 = Unbundle By Name(w1632) -> ("1  (A) cal"=w1625:dbl, "1 (V) cal"=w1624:dbl, "1 (PF) cal"=w1623:dbl, "2 (A) cal"=w1622:dbl, "2 (V) cal"=w1621:dbl, "2 (PF) cal"=w1620:dbl)  [unwired: 4 out]
                    n1013 = Multiply(x=w1631, y=w1625) -> (x*y=w1618:dbl)
                    n1014 = Multiply(x=w1630, y=w1624) -> (x*y=w1617:dbl)
                    n1015 = Multiply(x=w1629, y=w1623) -> (x*y=w1616:dbl)
                    n1016 = Multiply(x=w1628, y=w1622) -> (x*y=w1612:dbl)
                    n1017 = local read "LAB03-1 (SIG)"() -> (w1619:T2)
                    n1018 = Multiply(x=w1627, y=w1621) -> (x*y=w1611:dbl)
                    n1019 = Multiply(x=w1626, y=w1620) -> (x*y=w1610:dbl)
                    n1020 = local read "LAB03-1 (SIG)"() -> (w1614:T2)
                    n1021 = Bundle By Name(cluster=w1619, "AMPS"=w1618, "VOLTS"=w1617, "PF"=w1616) -> (w1615:T2)
                    n1022 = Bundle By Name(cluster=w1614, "AMPS"=w1612, "VOLTS"=w1611, "PF"=w1610) -> (w1613:T2)
                    n1023 = local write "LAB03-1 (SIG)"(w1613) -> ()
                    n1024 = local write "LAB03-1 (SIG)"(w1615) -> ()
                  }
                  frame #4 {
                    n1025 = local read "LAB04 (CAL)"() -> (w1656:T7)
                    n1026 = Unbundle By Name(w1633) -> ("LAB04-1 (A)"=w1655:dbl, "LAB04-1 (V)"=w1654:dbl, "LAB04-1 (PF)"=w1653:dbl, "LAB04-2 (A)"=w1652:dbl, "LAB04-2 (V)"=w1651:dbl, "LAB04-2 (PF)"=w1650:dbl)
                    n1027 = Unbundle By Name(w1656) -> ("1  (A) cal"=w1649:dbl, "1 (V) cal"=w1648:dbl, "1 (PF) cal"=w1647:dbl, "2 (A) cal"=w1646:dbl, "2 (V) cal"=w1645:dbl, "2 (PF) cal"=w1644:dbl)  [unwired: 4 out]
                    n1028 = Multiply(x=w1655, y=w1649) -> (x*y=w1642:dbl)
                    n1029 = Multiply(x=w1654, y=w1648) -> (x*y=w1641:dbl)
                    n1030 = Multiply(x=w1653, y=w1647) -> (x*y=w1640:dbl)
                    n1031 = Multiply(x=w1652, y=w1646) -> (x*y=w1636:dbl)
                    n1032 = local read "LAB04-1 (SIG)"() -> (w1643:T2)
                    n1033 = Multiply(x=w1651, y=w1645) -> (x*y=w1635:dbl)
                    n1034 = Multiply(x=w1650, y=w1644) -> (x*y=w1634:dbl)
                    n1035 = local read "LAB04-2 (SIG)"() -> (w1638:T2)
                    n1036 = Bundle By Name(cluster=w1643, "AMPS"=w1642, "VOLTS"=w1641, "PF"=w1640) -> (w1639:T2)
                    n1037 = Bundle By Name(cluster=w1638, "AMPS"=w1636, "VOLTS"=w1635, "PF"=w1634) -> (w1637:T2)
                    n1038 = local write "LAB04-2 (SIG)"(w1637) -> ()
                    n1039 = local write "LAB04-1 (SIG)"(w1639) -> ()
                  }
                  frame #5 {
                    n1040 = local read "LAB05 (CAL)"() -> (w1680:T7)
                    n1041 = Unbundle By Name(w1657) -> ("LAB05-1 (A)"=w1679:dbl, "LAB05-1 (V)"=w1678:dbl, "LAB05-1 (PF)"=w1677:dbl, "LAB05-2 (A)"=w1676:dbl, "LAB05-2 (V)"=w1675:dbl, "LAB05-2 (PF)"=w1674:dbl)
                    n1042 = Unbundle By Name(w1680) -> ("1  (A) cal"=w1673:dbl, "1 (V) cal"=w1672:dbl, "1 (PF) cal"=w1671:dbl, "2 (A) cal"=w1670:dbl, "2 (V) cal"=w1669:dbl, "2 (PF) cal"=w1668:dbl)  [unwired: 4 out]
                    n1043 = Multiply(x=w1679, y=w1673) -> (x*y=w1666:dbl)
                    n1044 = Multiply(x=w1678, y=w1672) -> (x*y=w1665:dbl)
                    n1045 = Multiply(x=w1677, y=w1671) -> (x*y=w1664:dbl)
                    n1046 = Multiply(x=w1676, y=w1670) -> (x*y=w1660:dbl)
                    n1047 = local read "LAB05-1 (SIG)"() -> (w1667:T2)
                    n1048 = Multiply(x=w1675, y=w1669) -> (x*y=w1659:dbl)
                    n1049 = Multiply(x=w1674, y=w1668) -> (x*y=w1658:dbl)
                    n1050 = local read "LAB05-2 (SIG)"() -> (w1662:T2)
                    n1051 = Bundle By Name(cluster=w1667, "AMPS"=w1666, "VOLTS"=w1665, "PF"=w1664) -> (w1663:T2)
                    n1052 = Bundle By Name(cluster=w1662, "AMPS"=w1660, "VOLTS"=w1659, "PF"=w1658) -> (w1661:T2)
                    n1053 = local write "LAB05-2 (SIG)"(w1661) -> ()
                    n1054 = local write "LAB05-1 (SIG)"(w1663) -> ()
                  }
                }
              }
            }
          }
          frame #12 {
            # "save test data to file"
            n1055 = local read "on loops"() -> (w1688:dbl)
            n1056 = local read "jig cycle"() -> (w1685:dbl)
            n1057 = Add(x=w1688, y=2) -> (x+y=w1686:dbl)
            n1058 = Equal?(x=w1685, y=1) -> (x = y?=w1683:bool)
            n1059 = Equal?(x=w1685, y=w1686) -> (x = y?=w1684:bool)
            n1060 = Or(x=w1683, y=w1684) -> (x .or. y?=w1682:bool)
            n1061 = case shown="True" w1682 {
              tunnel: w1681 -> [_ w1690]
              frame False {
              }
              frame True {
                n1062 = stacked-sequence {
                  tunnel: w1690 -> [w1691]
                  frame #0 {
                    # "LAB01-1"
                    n1063 = case shown="True" w1691 {
                      frame False {
                      }
                      frame True {
                        n1064 = local read "LAB01-1 (SIG)"() -> (w1734:T2)
                        n1065 = local read "LAB01 (DISP)"() -> (w1733:T5)
                        n1066 = local read "LAB01-1 (TDMS)"() -> (w1735:refnum<k34>)
                        n1067 = Build Array("TEMP Neut") -> (w1699:string[])
                        n1068 = Build Array("CYCLE") -> (w1694:string[])
                        n1069 = Build Array("TEMP Live") -> (w1704:string[])
                        n1070 = Build Array("PF") -> (w1709:string[])
                        n1071 = Build Array("AMPS") -> (w1730:string[])
                        n1072 = Build Array("VOLTS") -> (w1721:string[])
                        n1073 = Unbundle(w1734) -> ("AMPS"=w1729:dbl, "VOLTS"=w1718:dbl, "PF"=w1717:dbl, "Tmp Live"=w1716:dbl, "Tmp Neut"=w1719:dbl)
                        n1074 = Unbundle(w1733) -> ("1 (CYCLE)"=w1714:dbl)  [unwired: 5 out]
                        n1075 = Build Array(w1718) -> (w1715:dbl[])
                        n1076 = Build Array(w1717) -> (w1708:dbl[])
                        n1077 = Build Array(w1716) -> (w1703:dbl[])
                        n1078 = Build Array(w1719) -> (w1698:dbl[])
                        n1079 = Build Array(w1729) -> (w1728:dbl[])
                        n1080 = Build Array(w1714) -> (w1693:dbl[])
                        n1081 = TDMS Write(0:w1735, 5:"LAB01-1 TEST VALUES", 7:w1730, 9:w1728) -> (4:w1723:refnum<k34>, 6:w1722:string, 15:w1710:errorcluster)  [unwired: 2 in, 1 out]
                        n1082 = TDMS Write(0:w1723, 5:w1722, 7:w1721, 9:w1715, 11:w1710) -> (4:w1713:refnum<k34>, 6:w1712:string, 15:w1711:errorcluster)  [unwired: 1 in, 1 out]
                        n1083 = TDMS Write(0:w1713, 5:w1712, 7:w1709, 9:w1708, 11:w1711) -> (4:w1707:refnum<k34>, 6:w1706:string, 15:w1705:errorcluster)  [unwired: 1 in, 1 out]
                        n1084 = TDMS Write(0:w1707, 5:w1706, 7:w1704, 9:w1703, 11:w1705) -> (4:w1702:refnum<k34>, 6:w1701:string, 15:w1700:errorcluster)  [unwired: 1 in, 1 out]
                        n1085 = TDMS Write(0:w1702, 5:w1701, 7:w1699, 9:w1698, 11:w1700) -> (4:w1697:refnum<k34>, 6:w1696:string, 15:w1695:errorcluster)  [unwired: 1 in, 1 out]
                        n1086 = TDMS Write(0:w1697, 5:w1696, 7:w1694, 9:w1693, 11:w1695) -> (15:w1692:errorcluster)  [unwired: 1 in, 3 out]
                        n1087 = local write "data file error"(w1692) -> ()
                      }
                    }
                  }
                }
              }
            }
          }
          frame #13 {
            # "check for cycle test fail conditions"
            n1088 = local read "on loops"() -> (w1743:dbl)
            n1089 = local read "jig cycle"() -> (w1740:dbl)
            n1090 = local read "jig cycle"() -> (w1745:dbl)
            n1091 = Add(x=w1743, y=2.0) -> (x+y=w1741:dbl)
            n1092 = Equal?(x=w1745, y=1.0) -> (x = y?=w1738:bool)
            n1093 = Equal?(x=w1740, y=w1741) -> (x = y?=w1736:bool)
            n1094 = stacked-sequence {
              tunnel: w1739 -> [w1755]
              tunnel: w1738 -> [w1747]
              tunnel: w1737 -> [w1754]
              tunnel: w1736 -> [w1746]
              frame #0 {
                # "LAB01-1"
                n1095 = case shown="\"T-RISE TEST\"" w1755 {
                  tunnel: [FALSE TRUE FALSE] -> w1753
                  frame "TEST SET UP", Default {
                  }
                  frame "CYCLE TEST" {
                  }
                  frame "T-RISE TEST" {
                  }
                }
                n1096 = Or(x=w1747, y=w1746) -> (x .or. y?=w1751:bool)
                n1097 = local read "LAB01-1 (SIG)"() -> (w1749:T2)
                n1098 = And(x=w1754, y=w1751) -> (x .and. y?=w1750:bool)
                n1099 = Unbundle(w1749) -> ("AMPS"=w1748:dbl)  [unwired: 4 out]
                n1100 = And(x=w1753, y=w1750) -> (x .and. y?=w1752:bool)
                n1101 = stacked-sequence {
                  tunnel: w1752 -> [w1762]
                  tunnel: w1748 -> [w1761]
                  tunnel: w1747 -> [w1760]
                  tunnel: w1746 -> [w1759]
                  frame #0 {
                    n1102 = case shown="True" w1762 {
                      tunnel: w1761 -> [_ w1768]
                      tunnel: w1760 -> [_ w1770]
                      tunnel: w1759 -> [_ w1769]
                      frame False {
                      }
                      frame True {
                        # "check for amps fail"
                        n1103 = case shown="True" w1769 {
                          tunnel: w1768 -> [_ w1775]
                          tunnel: [FALSE w1774] -> w1766
                          tunnel: ["" "AMPS HI"] -> w1764
                          frame False {
                          }
                          frame True {
                            n1104 = Greater?(x=w1775, y=5.0) -> (0:w1774:bool)
                          }
                        }
                        n1105 = case shown="True" w1770 {
                          tunnel: w1768 -> [_ w1781]
                          tunnel: [FALSE w1780] -> w1767
                          tunnel: ["" "AMPS LO"] -> w1763
                          frame False {
                          }
                          frame True {
                            n1106 = Less?(x=w1781, y=5.0) -> (x < y?=w1780:bool)
                          }
                        }
                        n1107 = Or(x=w1767, y=w1766) -> (x .or. y?=w1765:bool)
                        n1108 = case shown="True" w1765 {
                          tunnel: w1764 -> [_ w1784]
                          tunnel: w1763 -> [_ w1783]
                          frame False {
                          }
                          frame True {
                            n1109 = stacked-sequence {
                              tunnel: w1784 -> [w1788 _]
                              tunnel: w1783 -> [w1787 _]
                              frame #0 {
                                n1110 = local read "LAB01-1 (TDMS)"() -> (w1791:refnum<k34>)
                                n1111 = Build Array(w1788, w1787) -> (w1786:string[])
                                n1112 = TDMS Write(0:w1791, 5:"TEST RESULT", 7:"AMPS FAIL ", 9:w1786) -> (15:w1790:errorcluster)  [unwired: 2 in, 3 out]
                                n1113 = local write "data file error"(w1790) -> ()
                              }
                              frame #1 {
                                n1114 = local read "LAB01 (DISP)"() -> (w1795:T5)
                                n1115 = Bundle(cluster=w1795, "1 (STATUS)"="STOP") -> (w1794:T5)  [unwired: 5 in]
                                n1116 = local write "LAB01-1 (RESULT)"(FALSE) -> ()
                                n1117 = local write "LAB01 (DISP)"(w1794) -> ()
                              }
                            }
                          }
                        }
                      }
                    }
                  }
                }
              }
            }
          }
          frame #14 {
            # "check for temperature rise test fail conditions"
            n1118 = stacked-sequence {
              tunnel: w1797 -> [w1817]
              tunnel: w1796 -> [w1816]
              frame #0 {
                # "LAB01-1"
                n1119 = local read "LAB01 (TEMP START)"() -> (w1810:T6)
                n1120 = local read "LAB01 (DISP)"() -> (w1801:T5)
                n1121 = local read "LAB01-1 (SIG)"() -> (w1812:T2)
                n1122 = local read "LAB01 (SET)"() -> (w1805:T4)
                n1123 = case shown="\"T-RISE TEST\"" w1817 {
                  tunnel: [FALSE FALSE TRUE] -> w1815
                  frame "TEST SET UP", Default {
                  }
                  frame "CYCLE TEST" {
                  }
                  frame "T-RISE TEST" {
                  }
                }
                n1124 = Unbundle(w1805) -> ("1 (T-RISE deg C)"=w1802:dbl)  [unwired: 9 out]
                n1125 = Unbundle(w1810) -> ("1 (TL)"=w1807:dbl, "1 (TN)"=w1806:dbl)  [unwired: 2 out]
                n1126 = Unbundle(w1801) -> ("1 (CYCLE)"=w1800:dbl)  [unwired: 5 out]
                n1127 = Unbundle(w1812) -> ("AMPS"=w1811:dbl, "Tmp Live"=w1809:dbl, "Tmp Neut"=w1808:dbl)  [unwired: 2 out]
                n1128 = Subtract(x=w1809, y=w1807) -> (x-y=w1804:dbl)
                n1129 = Greater?(x=w1800, y=2.0) -> (0:w1799:bool)
                n1130 = Subtract(x=w1808, y=w1806) -> (x-y=w1803:dbl)
                n1131 = And(x=w1816, y=w1799) -> (x .and. y?=w1813:bool)
                n1132 = And(x=w1815, y=w1813) -> (x .and. y?=w1814:bool)
                n1133 = case shown="True" w1814 {
                  tunnel: w1811 -> [_ w1833]
                  tunnel: w1804 -> [_ w1826]
                  tunnel: w1803 -> [_ w1825]
                  tunnel: w1802 -> [_ w1824]
                  frame False {
                  }
                  frame True {
                    # "check for amps & t-rise fail"
                    n1134 = Less?(x=w1833, y=5.0) -> (x < y?=w1819:bool)
                    n1135 = Greater?(x=w1826, y=w1824) -> (0:w1829:bool)
                    n1136 = Greater?(x=w1825, y=w1824) -> (0:w1830:bool)
                    n1137 = Or(x=w1829, y=w1830) -> (x .or. y?=w1818:bool)
                    n1138 = Select(t="AMPS LO", s=w1819, f="") -> (s? t:f=w1820:string)
                    n1139 = Select(t="T-RISE HI", s=w1818, f="") -> (s? t:f=w1821:string)
                    n1140 = Or(x=w1819, y=w1818) -> (x .or. y?=w1832:bool)
                    n1141 = case shown="True" w1832 {
                      tunnel: w1821 -> [_ w1835]
                      tunnel: w1820 -> [_ w1834]
                      frame False {
                      }
                      frame True {
                        n1142 = stacked-sequence {
                          tunnel: w1835 -> [w1837 _]
                          tunnel: w1834 -> [w1836 _]
                          frame #0 {
                            n1143 = local read "LAB01-1 (TDMS)"() -> (w1842:refnum<k34>)
                            n1144 = Build Array(w1836, w1837) -> (w1839:string[])
                            n1145 = TDMS Write(0:w1842, 5:"TEST RESULT", 7:"T-RISE FAIL ", 9:w1839) -> (15:w1841:errorcluster)  [unwired: 2 in, 3 out]
                            n1146 = local write "data file error"(w1841) -> ()
                          }
                          frame #1 {
                            n1147 = local read "LAB01 (DISP)"() -> (w1846:T5)
                            n1148 = Bundle(cluster=w1846, "1 (STATUS)"="STOP") -> (w1845:T5)  [unwired: 5 in]
                            n1149 = local write "LAB01-1 (RESULT)"(FALSE) -> ()
                            n1150 = local write "LAB01 (DISP)"(w1845) -> ()
                          }
                        }
                      }
                    }
                  }
                }
              }
            }
          }
          frame #15 {
            # "run calibration routine"
            n1151 = local read "CALIBRATE"() -> (w1850:bool)
            n1152 = case shown="True" w1850 {
              frame False {
              }
              frame True {
                n1153 = stacked-sequence {
                  seq-local: [w1851 _ _] -> [_ w1853 _]
                  frame #0 {
                    n1154 = call "CALIBRATION PASSWORD"() -> ("PASSWORD"=w1851:string)  [unwired: 17 in, 2 out]
                  }
                  frame #1 {
                    n1155 = Equal?(x=w1853, y="7777") -> (x = y?=w1852:bool)
                    n1156 = case shown="True" w1852 {
                      frame False {
                      }
                      frame True {
                        n1157 = stacked-sequence {
                          frame #0 {
                            n1158 = call "sub vi - calibration v1.vi"() -> ()  [unwired: 12 in]
                          }
                          frame #1 {
                            n1159 = call "sub vi - get calibration values v1.vi"() -> ("LAB01 (CAL)"=w1859:T7, "LAB02 (CAL)"=w1858:T8, "LAB03 (CAL)"=w1857:T7, "LAB04 (CAL)"=w1856:T7, "calibration file error out"=w1860:errorcluster, "LAB05 (CAL)"=w1855:T7)  [unwired: 10 in]
                            n1160 = local write "calibration file error out"(w1860) -> ()
                            n1161 = local write "LAB04 (CAL)"(w1856) -> ()
                            n1162 = local write "LAB05 (CAL)"(w1855) -> ()
                            n1163 = local write "LAB01 (CAL)"(w1859) -> ()
                            n1164 = local write "LAB02 (CAL)"(w1858) -> ()
                            n1165 = local write "LAB03 (CAL)"(w1857) -> ()
                          }
                        }
                      }
                    }
                  }
                  frame #2 {
                    n1166 = local write "CALIBRATE"(FALSE) -> ()
                  }
                }
              }
            }
          }
        }
        n1167 = node-c288() -> ()  [unwired: 1 in, 1 out]
        "loops" <- w33
      }
      n1168 = node-c288(w10) -> ()  [unwired: 1 out]
    }
  }
